vi "NEW数据采集传输系统.vi"() -> ()   [LabVIEW 2016, in "数据传输系统.lvlib"]
uses:
  <vilib>/Averna/Notify Icon/NotifyIcon.llb/BalloonIcon.ctl
  <vilib>/Utility/miscctls.llb/LVPointTypeDef.ctl
  <vilib>/Utility/config.llb/Read Key (String).vi
  <vilib>/Averna/Notify Icon/NotifyIcon.llb/GetSelectedItemEvent.vi
  <vilib>/Averna/Notify Icon/NotifyIcon.llb/SetVisible.vi
  <vilib>/Averna/Notify Icon/NotifyIcon.llb/SetMenuDefaultItem.vi
  <vilib>/Averna/Notify Icon/NotifyIcon.llb/SetTipText.vi
  <vilib>/Utility/config.llb/NI_LVConfig.lvlib
  data/FreeMem.dll
  <vilib>/Averna/Notify Icon/NotifyIcon.llb/NotifyIcon.lvclass
panel:
  out "错误输出":errorcluster
  in  "停止输入":bool caption="停止 2"
  in  "系统编码选择框":string(combo)="地表水质量监测"
  in  "数据发送通道":enum16{"TCP", "VISA"}(ring)
  in  "baud rate":u32=9600 caption="波特率"
  in  "VISA resource name":refnum<visa-resource-name> caption="VISA资源名称"
  in  "实时数据发送时间间隔/min":i32=1
  in  "数据组合发送":bool
  in  "日志、参数发送":bool
  in  "2011发送":bool
  in  "判断数据反馈":bool
  in  "数据发送协议":enum16{"2005-212协议", "2017-212协议"}(ring)=enum."2017-212协议"
  in  "重发时间":T1(ring)
  in  "重发日期":T2(ring)
  in  "开机启动":bool
  in  "确定更改起始时间":bool
  in  "更改起始时间":bool
  in  "数据发送起始时间":timestamp format="%<%.3X\n%Y/%m/%d>T"
  in  "每周自动重发":bool=TRUE
  in  "确定":bool
  in  "返回":bool
  in  "PW":string
  in  "MN":string
  in  "PORT":string
  in  "IP":string
  in  "站点设备":string
  in  "站点名称":string
  out "设置超时时间/min":i32=1
  out "状态信息":T3={"1st Error to Convert "=63, "步骤 "=enum."发送数据", "元素"="实时数据", "TCP服务端掉线计数"=0, "TCP掉线时间节点"="2019/05/08 15:24:17"} {"1st Error to Convert" items=["无错误", "参数错误", "内存已满", "超出区域", "文件结束", "文件已打开", "一般文件IO错误", "未找到文件", "文件权限错误", "磁盘已满", "路径副本", "打开过多文件", "未启用", "未找到资源文件", "无法添加资源", "未找到资源", "未找到图像", "图像内存错误", "画笔不存在", "配置错误类型", "配置未找到解析段", "配置解析错误", "配置内存错误", "错误外部代码格式", "错误外部代码偏移量", "外部代码不存在", "空窗口", "销毁窗口错误", "空菜单", "打印已中止", "错误打印记录", "打印驱动程序错误", "打印时窗口错误", "打印时内存错误", "打印对话框错误", "一般打印错误", "无效设备引用句柄", "设备未找到", "设备参数错误", "设备单位错误", "无法打开设备", "设备调用已中止", "一般错误", "用户已取消", "对象ID过低", "对象ID过高", "对象不在堆中", "未知的堆", "错误DefProc ID", "DefProc不在表格中", "范围外信息", "空方法", "未知信息", "不支持管理器调用", "错误地址", "连接过程中", "连接超时", "连接过程中", "不支持网络属性", "网络错误", "正在使用的地址", "系统缺少内存", "连接已中止", "连接已拒绝", "连接未建立", "连接已建立", "连接已关闭", "初始化错误（交互应用程序管理器）", "错误事件发生", "等待无约束事件发生处理程序", "事件发生队列溢出", "错误路径", "未发出信号量", "未识别类型（交互应用程序管理器）"]}
  out "数据接收超时指示灯":bool
  out "空闲时间/s":string
  out "系统时间":string
  out "实时小时数据上传":bool
  out "系统状态改变":bool
  out "软件版本":string
  out "掉线指示":bool
  out "核查数据上传":bool
  out "配置信息":T4
  in  "参数配置":bool
  out "查询数据发送":bool
  out "读取报文显示":string
  out "发送报文显示":string
  out "心跳包":bool
  out "通信状态":bool
  # "数 据 采 集 传 输 系 统"
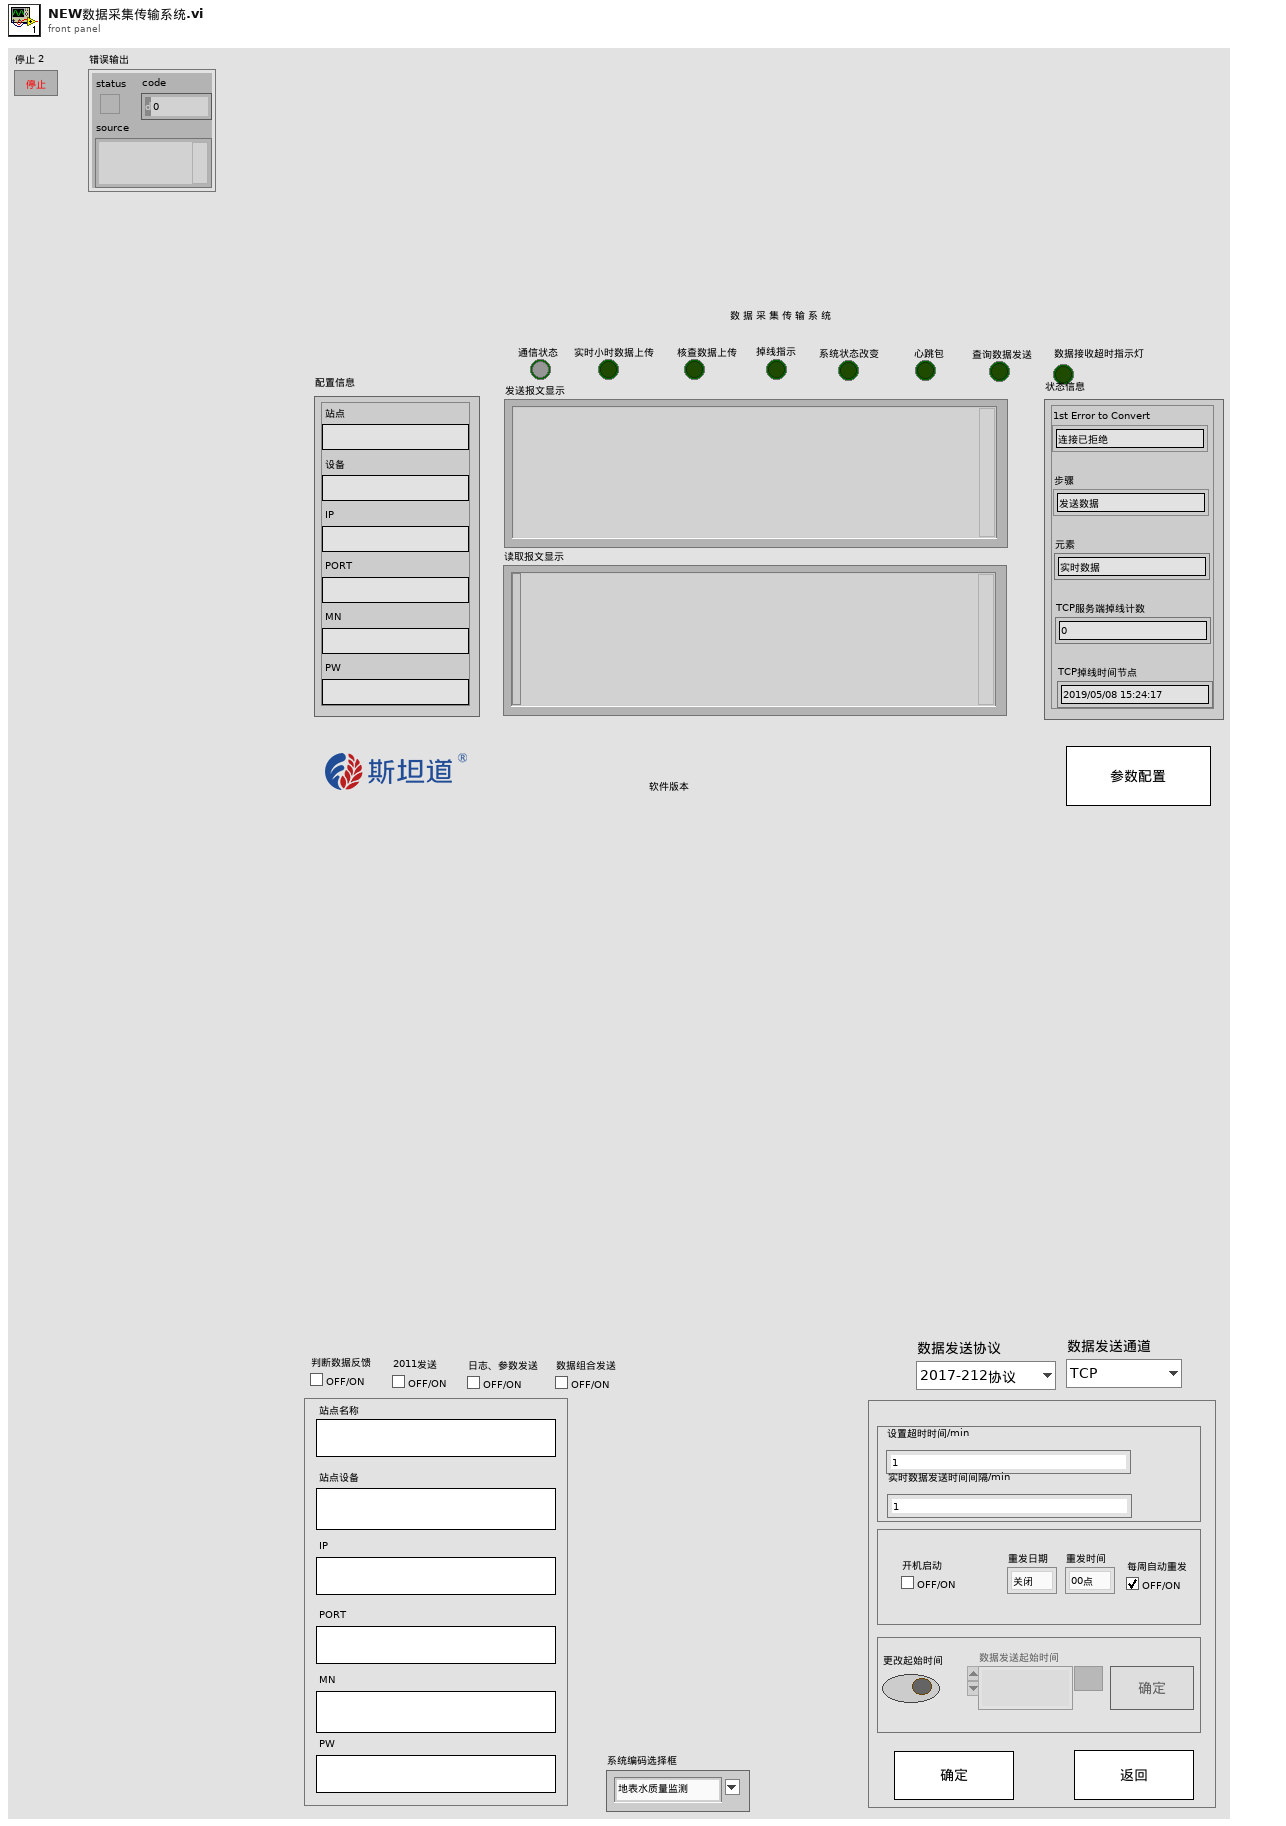
[diagram p1: front panel]
types:
  T1 = enum16{"00点", "01点", "02点", "03点", "04点", "05点", "06点", "07点", "08点", "09点", "10点", "11点", "12点", "13点", "14点", "15点", "16点", "17点", "18点", "19点", "20点", "21点", "22点", "23点"}
  T2 = enum16{"关闭", "星期日", "星期一", "星期二", "星期三", "星期四", "星期五", "星期六"}
  T3 = cluster{"1st Error to Convert ":i32, "步骤 ":enum16{"打开连接", "发送数据", "读取数据", "数据处理", "关闭连接"}, "元素":string, "TCP服务端掉线计数":i32, "TCP掉线时间节点":string}
  T4 = cluster{"站点":string, "设备":string, "IP":string, "PORT":string, "MN":string, "PW":string}
  T5 = enum32{"invalid app kind", "Development System", "Run Time System", "Student Edition", "Embedded LabVIEW", "Evaluation", "Custom"}
  T6 = enum8{"Enabled", "Disabled", "Disabled and Grayed Out"}
  T7 = typedef "LVPointTypeDef.ctl" = cluster{"Horizontal":i16, "Vertical":i16}
  T8 = typedef "imagedata.ctl" = cluster{"image type":i32, "image depth":i32, "image":u8[], "mask":u8[], "colors":u32[], "Rectangle":cluster{"left":i16, "top":i16, "right":i16, "bottom":i16}}
  T9 = typedef "NI_LVConfig.lvlib/Config Data RefNum.ctl" = refnum<k1>
  T10 = cluster{"CODMn":bool, "CODCr":bool, "DO":bool, "铜":bool, "PH":bool, "氨氮":bool, "比电导率":bool, "水温":bool, "盐度(海水)":bool, "浊度":bool, "总氮":bool, "总磷":bool, "叶绿素a":bool, "藻密度":bool, "水位":bool, "流速":bool, "瞬时流量":bool, "累积流量":bool}
  T11 = typedef "LVDateTimeRec.ctl" = cluster{"秒数的小数部分":dbl, "秒":i32, "分":i32, "时":i32, "日":i32, "月":i32, "年":i32, "天数（周）":i32, "天数（年）":i32, "DST":i32}
  T12 = enum32{"Invalid", "Standard", "Closed", "Hidden", "Minimized", "Maximized"}
  T13 = typedef "NotifyIcon.lvlib/NotifyIcon.lvclass/BalloonIcon.ctl" = enum32{"None", "Information", "Warning", "Error"}
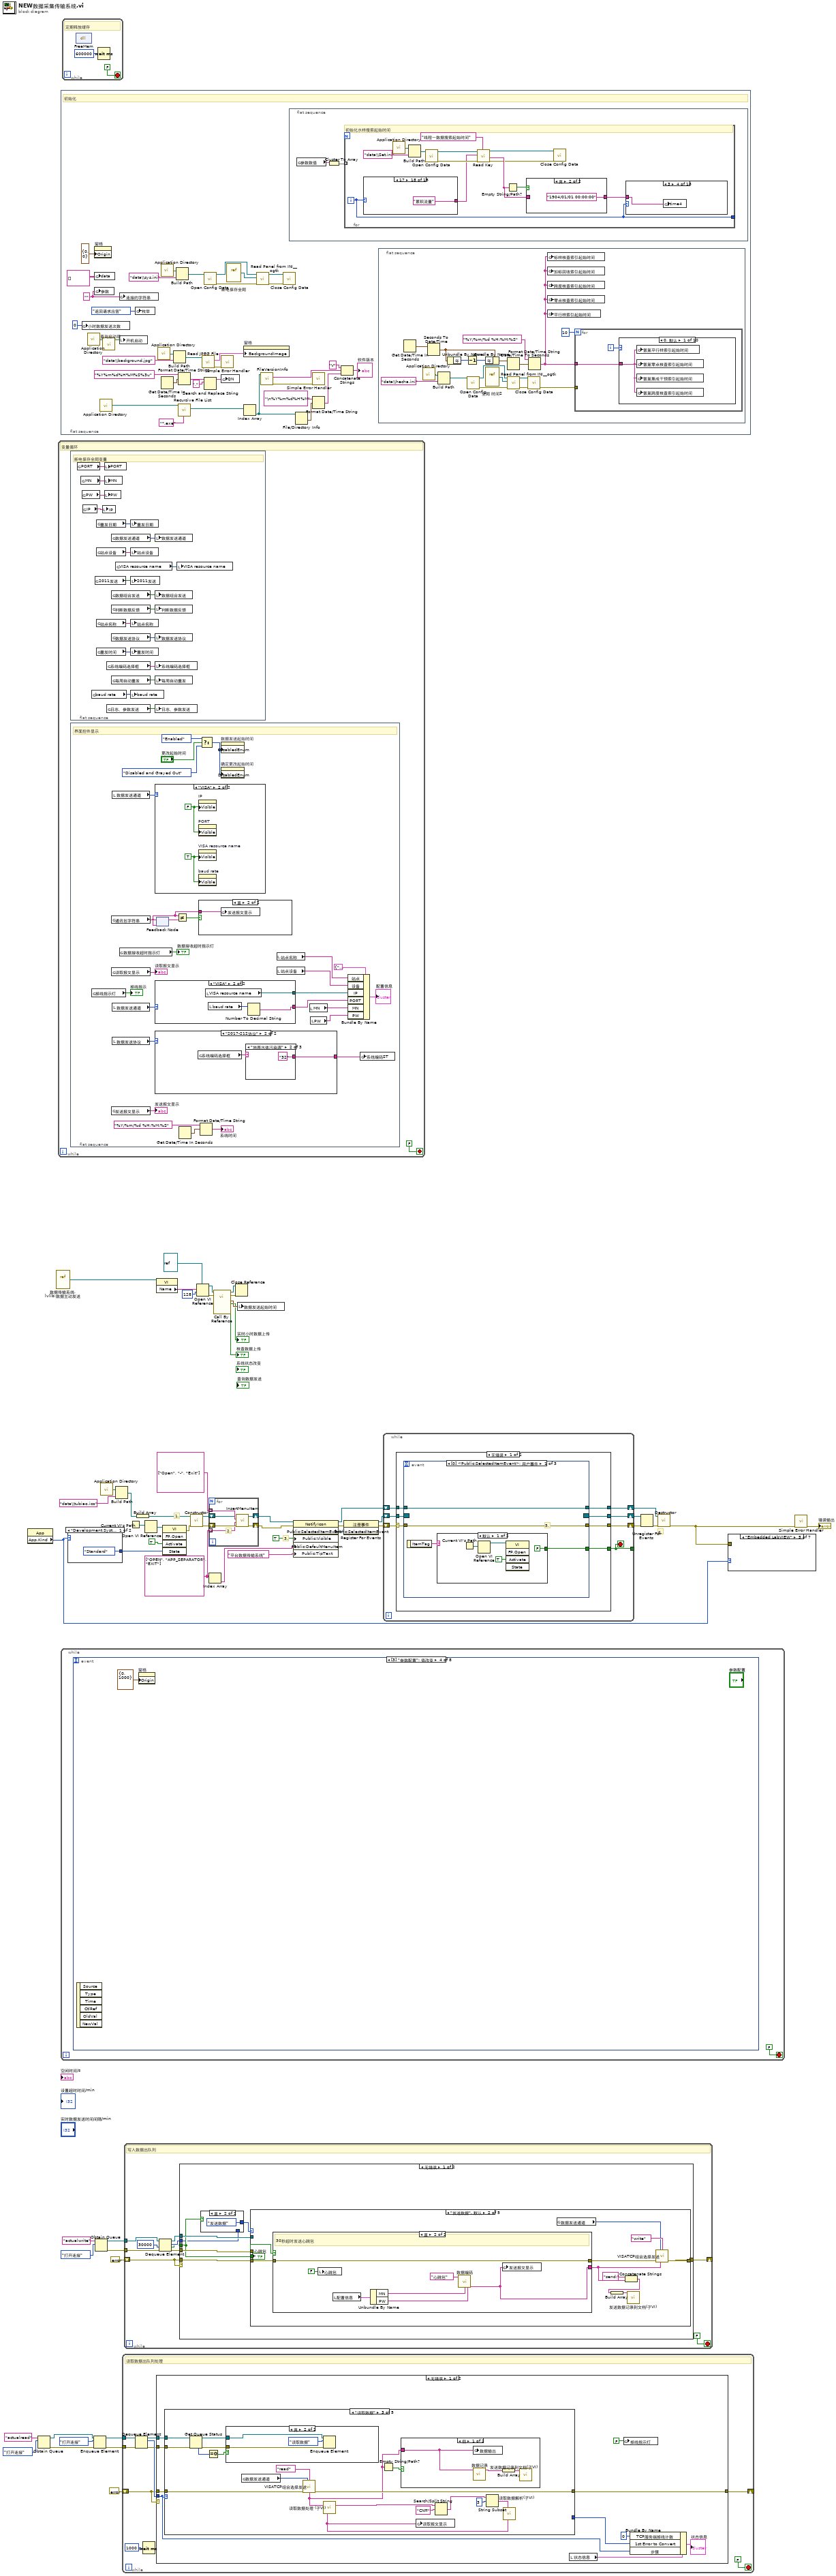
[diagram p0: block diagram]
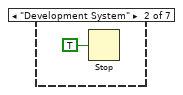
[diagram p3: hidden frame]
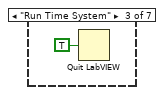
[diagram p4: hidden frame]
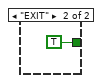
[diagram p8: hidden frame]
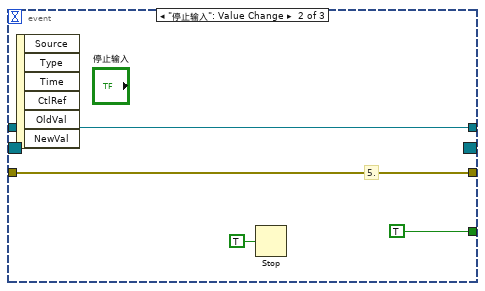
[diagram p9: hidden frame]
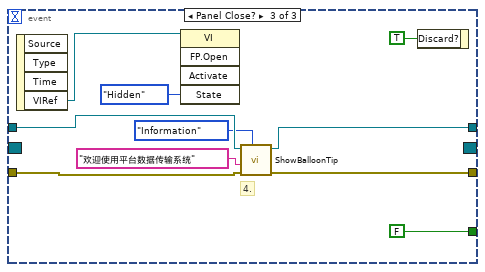
[diagram p10: hidden frame]
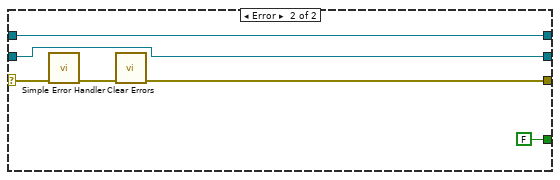
[diagram p11: hidden frame]
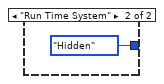
[diagram p12: hidden frame]
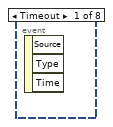
[diagram p13: hidden frame]
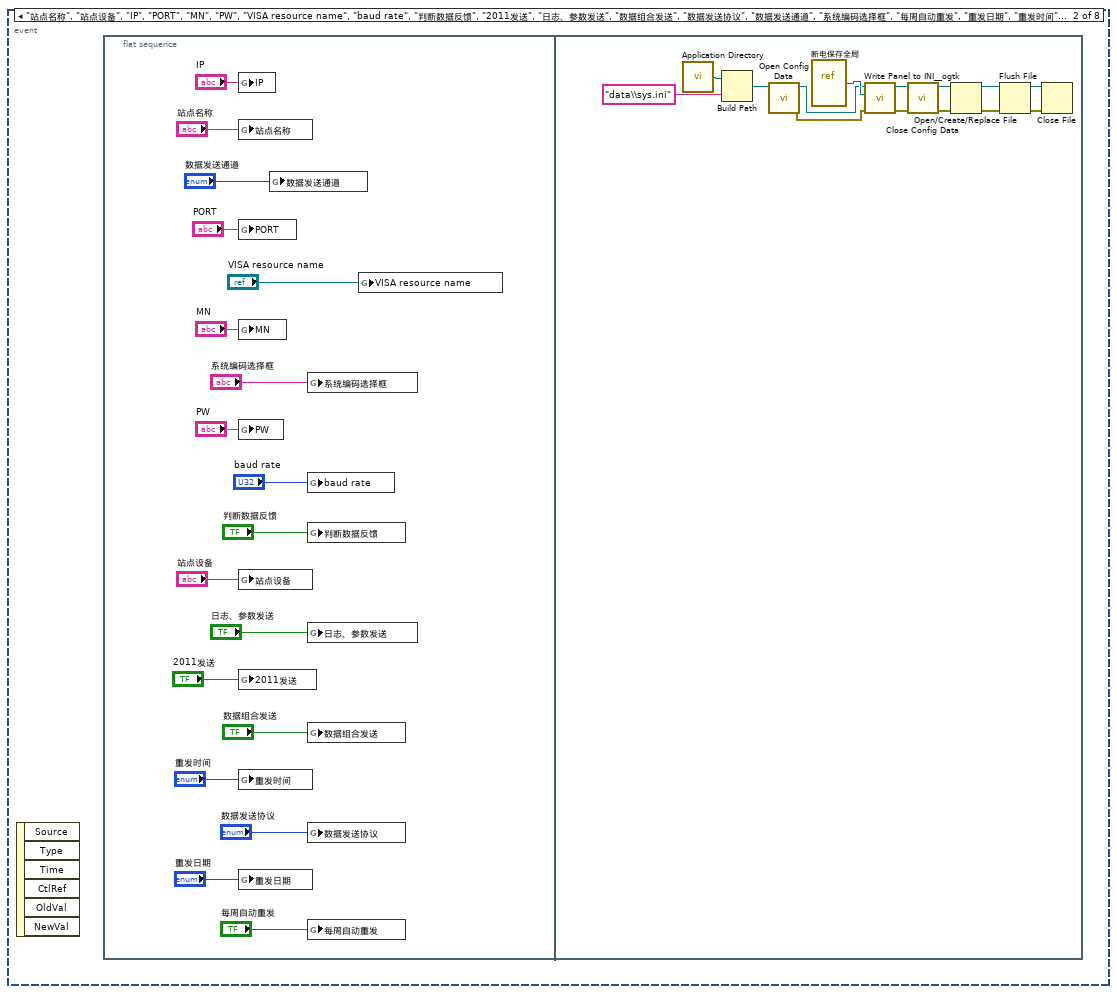
[diagram p14: hidden frame]
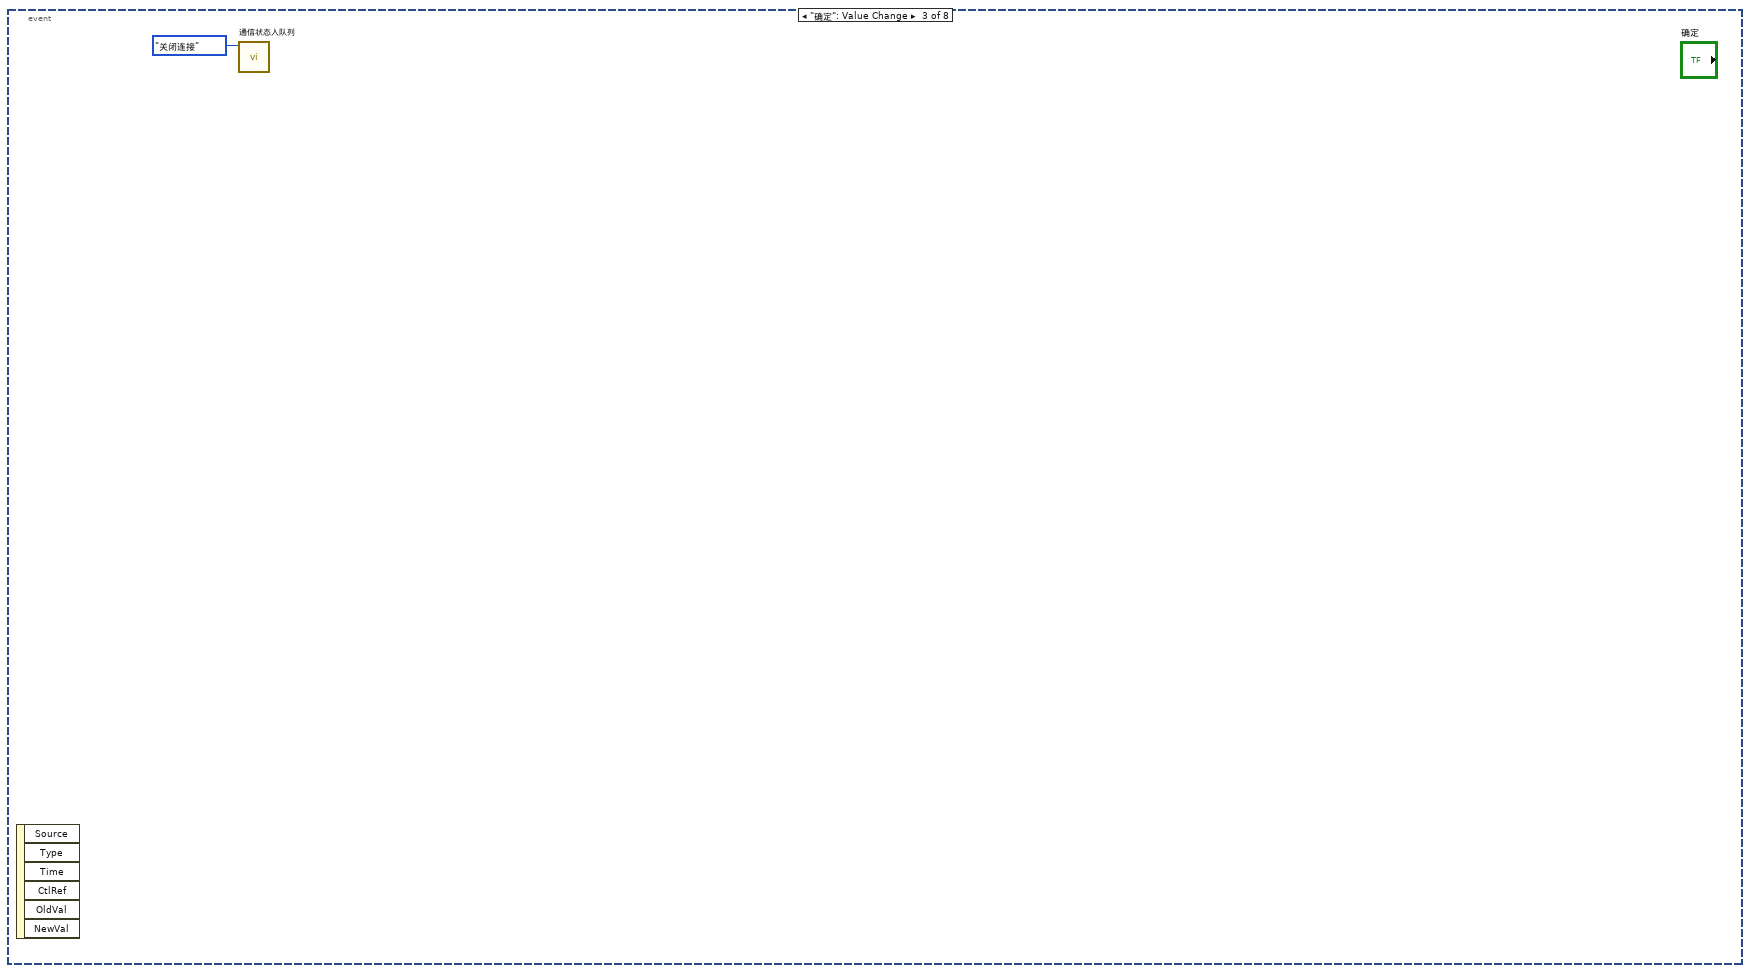
[diagram p15: hidden frame]
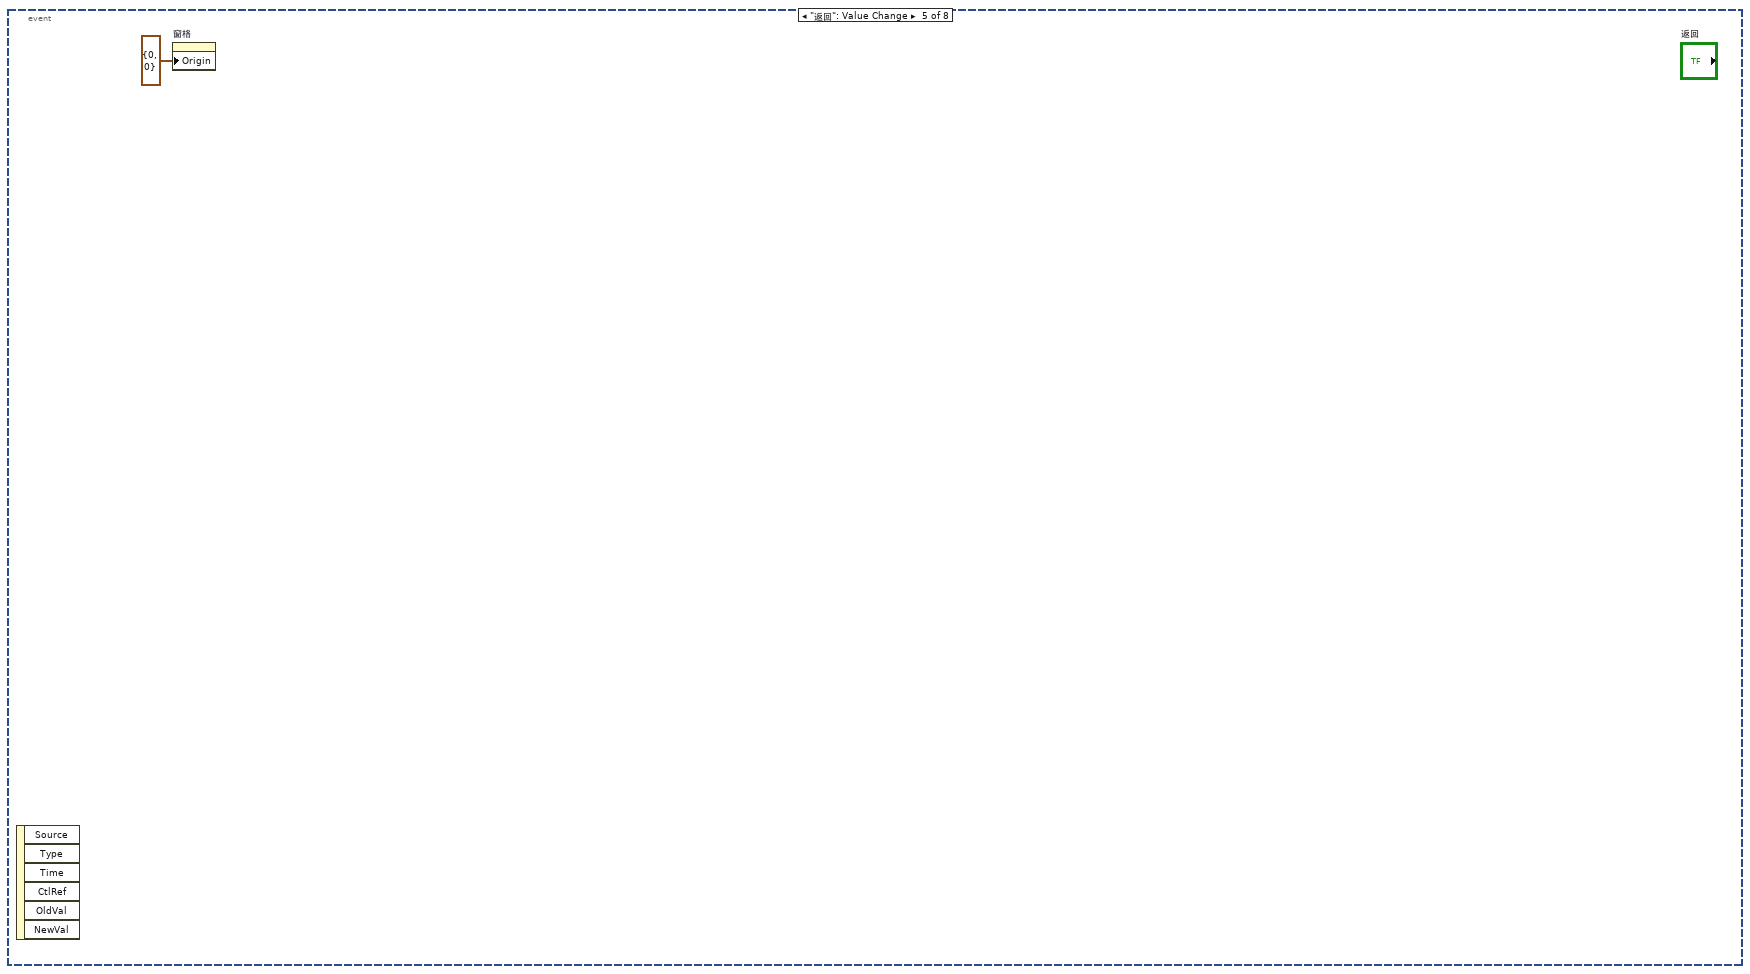
[diagram p16: hidden frame]
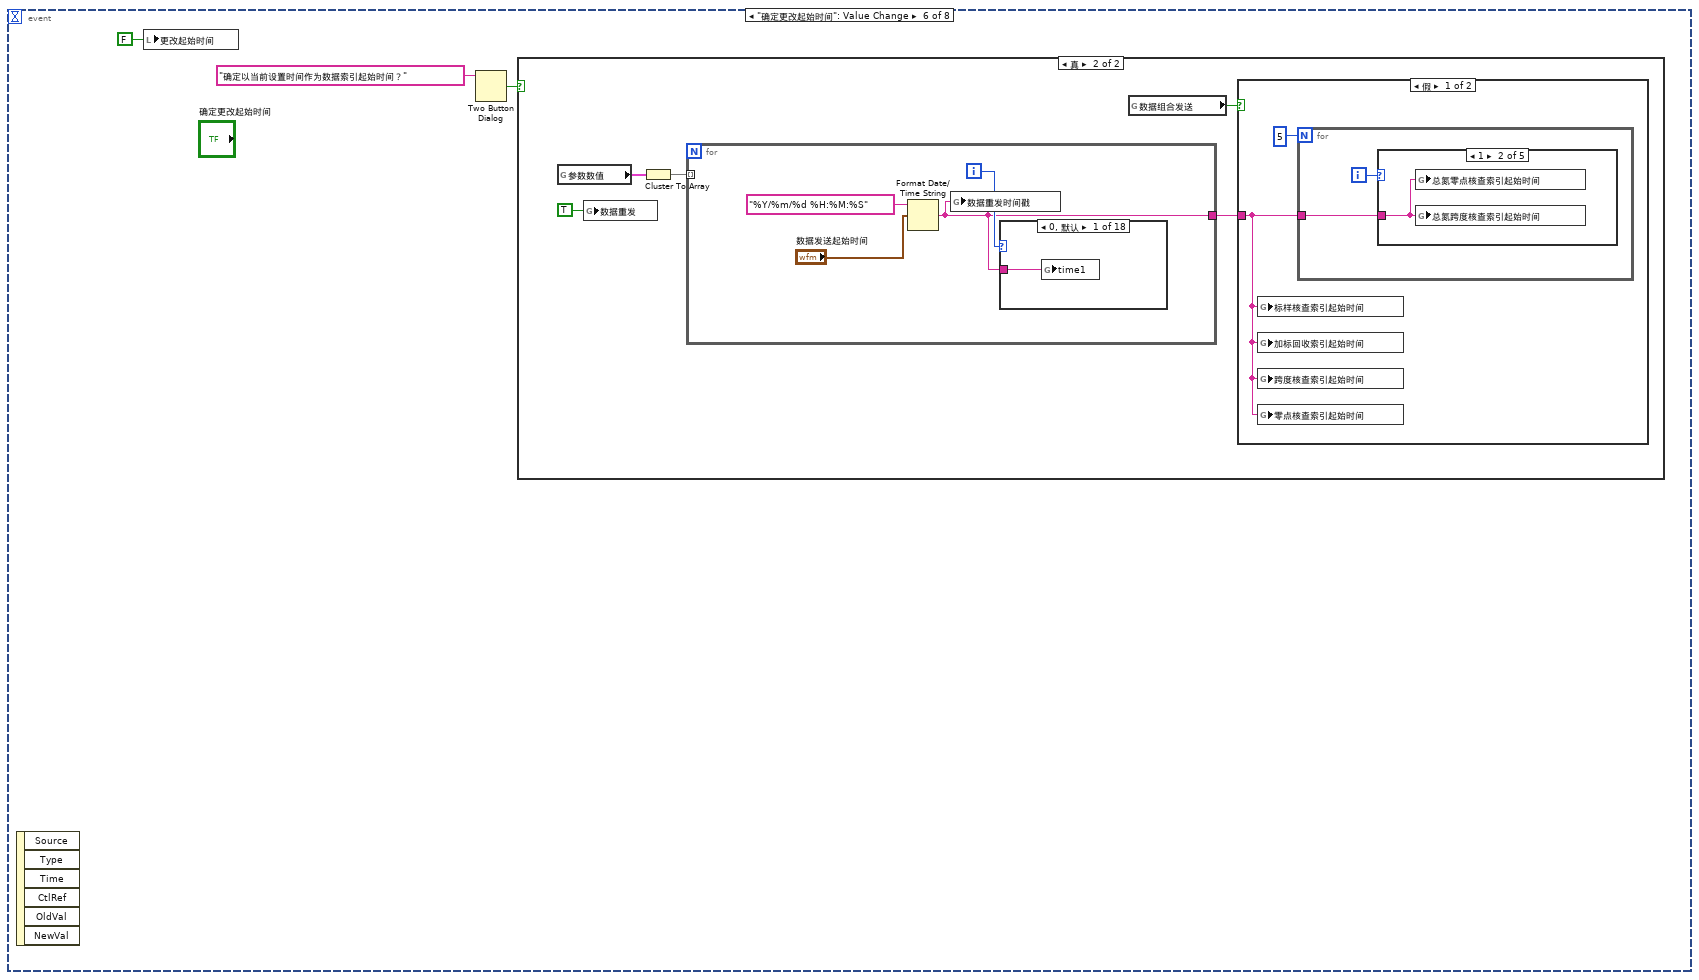
[diagram p17: hidden frame]
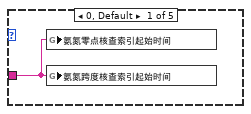
[diagram p19: hidden frame]
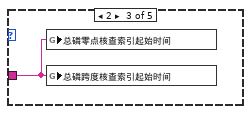
[diagram p20: hidden frame]
diagram:
  w9 = string[] ["OPEN", "APP_SEPARATOR", "EXIT"]
  # "6."
  # "3."
  # "1."
  n1 = property class="App"() -> ("App.Kind"=w1:T5)  [unwired: 2 in, 2 out]
  n2 = Obtain Queue(name (unnamed)="actualread" ("名称（未命名）"), element data type=enum16{"打开连接", "发送数据", "读取数据", "数据处理", "关闭连接"}."打开连接" ("枚举")) -> (queue out=w54:refnum<queue>, error out=w47:errorcluster)  [unwired: 3 in, 1 out]
  n3 = vi-ref "数据传输系统.lvlib:数据主动发送.vi"() -> (w41:refnum<vi>)
  n4 = while {
    stop <- FALSE stop-if-true
    # "变量循环"
    n5 = flat-sequence {
      frame #0 {
        # "断电保存全局变量"
        n6 = global read "断电保存全局.vi" "PORT"() -> (w112:string)
        n7 = global read "断电保存全局.vi" "MN"() -> (w111:string)
        n8 = global read "断电保存全局.vi" "PW"() -> (w110:string)
        n9 = global read "断电保存全局.vi" "IP"() -> (w113:string)
        n10 = global read "断电保存全局.vi" "baud rate"() -> (w108:u32)
        n11 = global read "断电保存全局.vi" "2011发送"() -> (w104:bool)
        n12 = global read "断电保存全局.vi" "重发日期"() -> (w106:T2)
        n13 = global read "断电保存全局.vi" "站点设备"() -> (w114:string)
        n14 = global read "断电保存全局.vi" "站点名称"() -> (w115:string)
        n15 = global read "断电保存全局.vi" "重发时间"() -> (w98:T1)
        n16 = local write "IP"(w113) -> ()
        n17 = local write "PORT"(w112) -> ()
        n18 = local write "MN"(w111) -> ()
        n19 = local write "PW"(w110) -> ()
        n20 = global read "断电保存全局.vi" "系统编码选择框"() -> (w99:string)
        n21 = global read "断电保存全局.vi" "日志、参数发送"() -> (w103:bool)
        n22 = global read "断电保存全局.vi" "数据发送通道"() -> (w100:enum16{"TCP", "VISA"})
        n23 = global read "断电保存全局.vi" "数据组合发送"() -> (w102:bool)
        n24 = global read "断电保存全局.vi" "判断数据反馈"() -> (w105:bool)
        n25 = global read "断电保存全局.vi" "数据发送协议"() -> (w101:enum16{"2005-212协议", "2017-212协议"})
        n26 = global read "断电保存全局.vi" "每周自动重发"() -> (w107:bool)
        n27 = global read "断电保存全局.vi" "VISA resource name"() -> (w109:refnum<visa-resource-name>)
        n28 = local write "重发日期"(w106) -> ()
        n29 = local write "站点设备"(w114) -> ()
        n30 = local write "2011发送"(w104) -> ()
        n31 = local write "站点名称"(w115) -> ()
        n32 = local write "重发时间"(w98) -> ()
        n33 = local write "baud rate"(w108) -> ()
        n34 = local write "数据发送通道"(w100) -> ()
        n35 = local write "数据组合发送"(w102) -> ()
        n36 = local write "判断数据反馈"(w105) -> ()
        n37 = local write "数据发送协议"(w101) -> ()
        n38 = local write "系统编码选择框"(w99) -> ()
        n39 = local write "每周自动重发"(w107) -> ()
        n40 = local write "日志、参数发送"(w103) -> ()
        n41 = local write "VISA resource name"(w109) -> ()
      }
    }
    n42 = flat-sequence {
      frame #0 {
        # "界面控件显示"
        n43 = global read "全局 数据发送重叠.vi" "掉线指示灯"() -> (→"掉线指示":bool)
        n44 = global read "全局1.vi" "通讯包字符串"() -> (w62:string)
        n45 = global read "全局1.vi" "读取报文显示"() -> (→"读取报文显示":string)
        n46 = global read "全局1.vi" "发送报文显示"() -> (→"发送报文显示":string)
        n47 = local read "数据发送通道"() -> (w56:enum16{"TCP", "VISA"})
        n48 = local read "数据发送通道"() -> (w81:enum16{"TCP", "VISA"})
        n49 = local read "数据发送协议"() -> (w70:enum16{"2005-212协议", "2017-212协议"})
        n50 = global read "全局 数据发送重叠.vi" "数据接收超时指示灯"() -> (→"数据接收超时指示灯":bool)
        n51 = case shown="\"VISA\"" w56 {
          frame "TCP", Default {
            w82 = TRUE ("可见")
            w83 = FALSE ("可见")
            n52 = property on="IP" class="Str"("Visible"=w82) -> ()  [unwired: 2 in, 2 out]
            n53 = property on="PORT" class="Str"("Visible"=w82) -> ()  [unwired: 2 in, 2 out]
            n54 = property on="VISA resource name" class="VISAName"("Visible"=w83) -> ()  [unwired: 2 in, 2 out]
            n55 = property on="baud rate" class="DigNum (严格)"("Visible"=w83) -> ()  [unwired: 2 in, 2 out]
          }
          frame "VISA" {
            w84 = FALSE ("可见")
            w85 = TRUE ("可见")
            n56 = property on="IP" class="Str"("Visible"=w84) -> ()  [unwired: 2 in, 2 out]
            n57 = property on="PORT" class="Str"("Visible"=w84) -> ()  [unwired: 2 in, 2 out]
            n58 = property on="VISA resource name" class="VISAName"("Visible"=w85) -> ()  [unwired: 2 in, 2 out]
            n59 = property on="baud rate" class="DigNum (严格)"("Visible"=w85) -> ()  [unwired: 2 in, 2 out]
          }
        }
        n60 = case shown="\"VISA\"" w81 {
          tunnel: [w94 w97] -> w78
          tunnel: [w93 w95] -> w75
          frame "TCP", Default {
            n61 = local read "PORT"() -> (w93:string)
            n62 = local read "IP"() -> (w94:string)
          }
          frame "VISA" {
            n63 = local read "VISA resource name"() -> (w97:refnum<visa-resource-name>)
            n64 = local read "baud rate"() -> (w96:u32)
            n65 = Number To Decimal String(number=w96) -> (decimal integer string=w95:string)  [unwired: 1 in]
          }
        }
        n66 = case shown="\"2017-212协议\"" w70 {
          tunnel: ["32" ("设备编码MN") w88] -> w69
          frame "2005-212协议", Default {
          }
          frame "2017-212协议" {
            n67 = global read "断电保存全局.vi" "系统编码选择框"() -> (w89:string)
            n68 = case shown="\"地表水体污染源\"" w89 {
              tunnel: ["52" ("设备编码MN") "32" ("设备编码MN") "21" ("设备编码MN")] -> w88
              frame "污水排放过程监测" {
              }
              frame "地表水体污染源" {
              }
              frame "地表水质量监测", Default {
              }
            }
          }
        }
        n69 = feedback #1(w62) -> (w63:string)
        n70 = feedback-in #1(w62) -> ()
        n71 = Not Equal?(x=w62, y=w63) -> (x != y?=w61:bool)
        n72 = Get Date/Time In Seconds() -> (seconds since 1Jan1904=w71:timestamp)
        n73 = case shown="真" w61 {
          tunnel: w62 -> [_ w86]
          frame False {
          }
          frame True {
            n74 = global write "全局1.vi" "发送报文显示"(w86) -> ()
          }
        }
        n75 = Format Date/Time String(time format string (%c)="%Y/%m/%d %H:%M:%S" ("时间格式字符串(%c)"), seconds (now)=w71) -> (date/time string=→"系统时间":string)  [unwired: 1 in]
        n76 = Select(t=T6."Enabled" ("禁用"), s="更改起始时间", f=T6."Disabled and Grayed Out" ("禁用")) -> (s? t:f=w57:T6)
        n77 = property on="数据发送起始时间" class="AbsTime (严格)"("DisabledEnum"=w57) -> ()  [unwired: 2 in, 2 out]
        n78 = property on="确定更改起始时间" class="Bool"("DisabledEnum"=w57) -> ()  [unwired: 2 in, 2 out]
        n79 = local read "站点名称"() -> (w77:string)
        n80 = local read "站点设备"() -> (w76:string)
        n81 = local read "MN"() -> (w74:string)
        n82 = local read "PW"() -> (w73:string)
        n83 = Bundle By Name(cluster=T4 {"站点"="", "设备"="", "IP"="", "PORT"="", "MN"="", "PW"=""} ("配置信息"), "站点"=w77, "设备"=w76, "IP"=w78, "PORT"=w75, "MN"=w74, "PW"=w73) -> (→"配置信息":T4)
        n84 = global write "全局1.vi" "系统编码ST"(w69) -> ()
      }
    }
  }
  n85 = flat-sequence {
    frame #0 {
      w149 = "" ("参数")
      # "初始化"
      n86 = global write "全局 小时数据发送次数.vi" "小时数据发送次数"(0 ("数值")) -> ()
      n87 = call <vilib>:"Application Directory.vi"() -> ("Application Directory"=w125:path)
      n88 = property on="窗格" class="Pane"("Origin"=T7 {"Horizontal"=0, "Vertical"=0} ("原点")) -> ()  [unwired: 2 in, 2 out]
      n89 = global write "全局 实时数据参数.vi" "data"(string[][] [] ("data")) -> ()
      n90 = global write "全局 实时数据参数.vi" "参数"(w149) -> ()
      n91 = call <vilib>:"Application Directory.vi"() -> ("Application Directory"=w128:path)
      n92 = call "查询启动项.vi"("启动文件路径"=w125) -> ("包含启动项"=w124:bool)  [unwired: 9 in, 1 out]
      n93 = global write "全局 实时数据参数.vi" "连接的字符串"(w149) -> ()
      n94 = local write "开机启动"(w124) -> ()
      n95 = global write "全局1.vi" "枚举"(enum16{"返回请求应答", "上传数据", "返回执行结果"}."返回请求应答" ("枚举")) -> ()
      n96 = call <vilib>:"Application Directory.vi"() -> ("Application Directory"=w140:path)
      n97 = call <vilib>:"Application Directory.vi"() -> ("Application Directory"=w119:path)
      n98 = Get Date/Time In Seconds() -> (seconds since 1Jan1904=w145:timestamp)
      n99 = Build Path(base path=w140, name or relative path="data\\background.jpg" ("名称或相对路径")) -> (appended path=w139:path)
      n100 = Build Path(base path=w119, name or relative path="data\\sys.ini" ("名称或相对路径")) -> (appended path=w117:path)
      n101 = Format Date/Time String(time format string (%c)="%Y%m%d%H%M%S%3u" ("时间格式字符串(%c)"), seconds (now)=w145) -> (date/time string=w144:string)  [unwired: 1 in]
      n102 = call <vilib>:"Recursive File List.vi"("pattern"="*.exe", "Folder Path"=w128) -> ("All Files in Dir"=w135:path[])  [unwired: 5 in, 4 out]
      n103 = call <vilib>:"Read JPEG File.vi"("path to JPEG file"=w139) -> ("error out"=w137:errorcluster, "image data"=w138:T8)  [unwired: 8 in, 1 out]
      n104 = call <vilib>:"Open Config Data.vi"("configuration file path"=w117) -> ("error out"=w123:errorcluster, "refnum"=w122:T9)  [unwired: 8 in, 1 out]
      n105 = Search and Replace String(input string=w144, search string="." ("搜索字符串")) -> (result string=w142:string)  [unwired: 6 in, 3 out]
      n106 = call <vilib>:"Simple Error Handler.vi"("error in (no error)"=w137) -> ()  [unwired: 4 in, 5 out]
      n107 = global write "全局1.vi" "QN"(w142) -> ()
      n108 = vi-ref "断电保存全局.vi"() -> (w121:refnum<vi>)
      n109 = property on="窗格" class="Pane"("BackgroundImage"=w138) -> ()  [unwired: 2 in, 2 out]
      n110 = Index Array(array=w135) -> (element=w134:path)  [unwired: 1 in]
      n111 = call <userlib>:"Read Panel from INI__ogtk.vi"("error in (no error)"=w123, "VI ref"=w121, "refnum"=w122) -> ("error out"=w116:errorcluster, "refnum out"=w120:T9)  [unwired: 7 in]
      n112 = call <vilib>:"FileVersionInfo.vi"("Application Path in"=w134) -> ("error out"=w127:errorcluster, "File Version Info"=w130:string)  [unwired: 7 in, 2 out]
      n113 = call <vilib>:"Close Config Data.vi"("error in (no error)"=w116, "refnum"=w120) -> ()  [unwired: 8 in, 2 out]
      n114 = flat-sequence {
        frame #0 {
          n115 = global read "全局1.vi" "参数数值"() -> (w152:T10)
          n116 = Cluster To Array(cluster=w152) -> (array=w153:bool[])
          n117 = for {
            tunnel: w153 -> [_] mode=indexing
            tunnel: [w156] -> _
            i -> [w156]
            # "初始化水样搜索起始时间"
            n118 = case shown="17" w156 {
              tunnel: ["CODMn" "CODCr" "DO" "铜" "PH" "氨氮" "比电导率" "水温" "盐度(海水)" "浊度" "总氮" "总磷" "叶绿素a" "藻密度" "水位" "流速" "瞬时流量" "累积流量"] -> w160
              frame 0, Default {
              }
              frame 1 {
              }
              frame 2 {
              }
              frame 3 {
              }
              frame 4 {
              }
              frame 5 {
              }
              frame 6 {
              }
              frame 7 {
              }
              frame 8 {
              }
              frame 9 {
              }
              frame 10 {
              }
              frame 11 {
              }
              frame 12 {
              }
              frame 13 {
              }
              frame 14 {
              }
              frame 15 {
              }
              frame 16 {
              }
              frame 17 {
              }
            }
            n119 = call <vilib>:"Application Directory.vi"() -> ("Application Directory"=w166:path)
            n120 = Build Path(base path=w166, name or relative path="data\\Set.ini" ("名称或相对路径")) -> (appended path=w164:path)
            n121 = call <vilib>:"Open Config Data.vi"("configuration file path"=w164) -> ("error out"=w162:errorcluster, "refnum"=w163:T9)  [unwired: 8 in, 1 out]
            n122 = call-poly <vilib>:"Read Key.vi"("section"="线程一数据搜索起始时间", "error in (no error)"=w162, "key"=w160, "refnum"=w163) -> ("error out"=w154:errorcluster, "value"=w157:string, "refnum out"=w155:T9)  [unwired: 4 in, 1 out]
            n123 = Empty String/Path?(string/path=w157) -> (empty?=w159:bool)
            n124 = case shown="真" w159 {
              tunnel: [w167 "1904/01/01 00:00:00"] -> w158
              tunnel: w157 -> [w167 _]
              frame False {
              }
              frame True {
              }
            }
            n125 = call <vilib>:"Close Config Data.vi"("error in (no error)"=w154, "refnum"=w155) -> ()  [unwired: 8 in, 2 out]
            n126 = case shown="3" w156 {
              tunnel: w158 -> [w169 w170 w171 w172 w173 w174 w175 w176 w177 w178 w179 w180 w181 w182 w183 w184 w185 w186]
              frame 0, Default {
                n127 = global write "全局 水样时间.vi" "time1"(w169) -> ()
              }
              frame 1 {
                n128 = global write "全局 水样时间.vi" "time2"(w170) -> ()
              }
              frame 2 {
                n129 = global write "全局 水样时间.vi" "time3"(w171) -> ()
              }
              frame 3 {
                n130 = global write "全局 水样时间.vi" "time4"(w172) -> ()
              }
              frame 4 {
                n131 = global write "全局 水样时间.vi" "time5"(w173) -> ()
              }
              frame 5 {
                n132 = global write "全局 水样时间.vi" "time6"(w174) -> ()
              }
              frame 6 {
                n133 = global write "全局 水样时间.vi" "time7"(w175) -> ()
              }
              frame 7 {
                n134 = global write "全局 水样时间.vi" "time8"(w176) -> ()
              }
              frame 8 {
                n135 = global write "全局 水样时间.vi" "time9"(w177) -> ()
              }
              frame 9 {
                n136 = global write "全局 水样时间.vi" "time10"(w178) -> ()
              }
              frame 10 {
                n137 = global write "全局 水样时间.vi" "time11"(w179) -> ()
              }
              frame 11 {
                n138 = global write "全局 水样时间.vi" "time12"(w180) -> ()
              }
              frame 12 {
                n139 = global write "全局 水样时间.vi" "time13"(w181) -> ()
              }
              frame 13 {
                n140 = global write "全局 水样时间.vi" "time14"(w182) -> ()
              }
              frame 14 {
                n141 = global write "全局 水样时间.vi" "time15"(w183) -> ()
              }
              frame 15 {
                n142 = global write "全局 水样时间.vi" "time16"(w184) -> ()
              }
              frame 16 {
                n143 = global write "全局 水样时间.vi" "time17"(w185) -> ()
              }
              frame 17 {
                n144 = global write "全局 水样时间.vi" "time18"(w186) -> ()
              }
            }
          }
        }
      }
      n145 = File/Directory Info(path=w134) -> (last mod=w133:timestamp)  [unwired: 1 in, 6 out]
      n146 = call <vilib>:"Simple Error Handler.vi"("error in (no error)"=w127) -> ()  [unwired: 4 in, 5 out]
      n147 = Format Date/Time String(time format string (%c)="\n%Y%m%d%H%M" ("时间格式字符串(%c)"), seconds (now)=w133) -> (date/time string=w129:string)  [unwired: 1 in]
      n148 = Concatenate Strings("V" ("字符串"), w130, w129) -> (→"软件版本":string)
      n149 = flat-sequence {
        frame #0 {
          n150 = Get Date/Time In Seconds() -> (seconds since 1Jan1904=w222:timestamp)
          n151 = call <vilib>:"Application Directory.vi"() -> ("Application Directory"=w212:path)
          n152 = Seconds To Date/Time(time stamp (now)=w222) -> (date time rec=w220:T11)  [unwired: 1 in]
          n153 = Build Path(base path=w212, name or relative path="data\\hecha.ini" ("名称或相对路径")) -> (appended path=w214:path)
          n154 = Unbundle By Name(w220) -> ("年"=w221:i32)
          n155 = Decrement(x=w221) -> (x-1=w219:i32)
          n156 = call <vilib>:"Open Config Data.vi"("configuration file path"=w214) -> ("error out"=w208:errorcluster, "refnum"=w209:T9)  [unwired: 8 in, 1 out]
          n157 = Bundle By Name(cluster=w220, "年"=w219) -> (w217:T11)
          n158 = vi-ref "全局 时间2.vi"() -> (w210:refnum<vi>)
          n159 = Date/Time To Seconds(2:w217) -> (0:w218:timestamp)  [unwired: 1 in]
          n160 = call <userlib>:"Read Panel from INI__ogtk.vi"("error in (no error)"=w208, "VI ref"=w210, "refnum"=w209) -> ("error out"=w207:errorcluster, "refnum out"=w211:T9)  [unwired: 7 in]
          n161 = call <vilib>:"Close Config Data.vi"("error in (no error)"=w207, "refnum"=w211) -> ("error out"=w206:errorcluster)  [unwired: 8 in, 1 out]
          n162 = Format Date/Time String(time format string (%c)="%Y/%m/%d %H:%M:%S" ("时间格式字符串(%c)"), seconds (now)=w218) -> (date/time string=w215:string)  [unwired: 1 in]
          n163 = global write "全局 时间2.vi" "标样核查索引起始时间"(w215) -> ()
          n164 = global write "全局 时间2.vi" "加标回收索引起始时间"(w215) -> ()
          n165 = global write "全局 时间2.vi" "跨度核查索引起始时间"(w215) -> ()
          n166 = global write "全局 时间2.vi" "零点核查索引起始时间"(w215) -> ()
          n167 = global write "全局 时间2.vi" "平行样索引起始时间"(w215) -> ()
          n168 = for {
            N: 10 -> [_]
            tunnel: w215 -> [w223]
            tunnel: w206 -> [_]
            i -> [w224]
            n169 = case shown="0, 默认" w224 {
              tunnel: w223 -> [w225 w226 w227 w228 w229 w230 w231 w232 w233 w234]
              frame 0, Default {
                n170 = global write "全局 时间2.vi" "氨氮平行样索引起始时间"(w225) -> ()
                n171 = global write "全局 时间2.vi" "氨氮零点核查索引起始时间"(w225) -> ()
                n172 = global write "全局 时间2.vi" "氨氮集成干预索引起始时间"(w225) -> ()
                n173 = global write "全局 时间2.vi" "氨氮跨度核查索引起始时间"(w225) -> ()
              }
              frame 1 {
                n174 = global write "全局 时间2.vi" "总氮零点核查索引起始时间"(w226) -> ()
                n175 = global write "全局 时间2.vi" "总氮平行样索引起始时间"(w226) -> ()
                n176 = global write "全局 时间2.vi" "总氮跨度核查索引起始时间"(w226) -> ()
                n177 = global write "全局 时间2.vi" "总氮集成干预索引起始时间"(w226) -> ()
              }
              frame 2 {
                n178 = global write "全局 时间2.vi" "总磷零点核查索引起始时间"(w227) -> ()
                n179 = global write "全局 时间2.vi" "总磷平行样索引起始时间"(w227) -> ()
                n180 = global write "全局 时间2.vi" "总磷跨度核查索引起始时间"(w227) -> ()
                n181 = global write "全局 时间2.vi" "总磷集成干预索引起始时间"(w227) -> ()
              }
              frame 3 {
                n182 = global write "全局 时间2.vi" "CODMn零点核查索引起始时间"(w228) -> ()
                n183 = global write "全局 时间2.vi" "CODMn平行样索引起始时间"(w228) -> ()
                n184 = global write "全局 时间2.vi" "CODMn跨度核查索引起始时间"(w228) -> ()
                n185 = global write "全局 时间2.vi" "CODMn集成干预索引起始时间"(w228) -> ()
              }
              frame 4 {
                n186 = global write "全局 时间2.vi" "CODCr零点核查索引起始时间"(w229) -> ()
                n187 = global write "全局 时间2.vi" "CODCr平行样索引起始时间"(w229) -> ()
                n188 = global write "全局 时间2.vi" "CODCr跨度核查索引起始时间"(w229) -> ()
                n189 = global write "全局 时间2.vi" "CODCr集成干预索引起始时间"(w229) -> ()
              }
              frame 5 {
                n190 = global write "全局 时间2.vi" "DO集成干预索引起始时间"(w230) -> ()
              }
              frame 6 {
                n191 = global write "全局 时间2.vi" "PH集成干预索引起始时间"(w231) -> ()
              }
              frame 7 {
                n192 = global write "全局 时间2.vi" "比电导率集成干预索引起始时间"(w232) -> ()
              }
              frame 8 {
                n193 = global write "全局 时间2.vi" "水温集成干预索引起始时间"(w233) -> ()
              }
              frame 9 {
                n194 = global write "全局 时间2.vi" "浊度集成干预索引起始时间"(w234) -> ()
              }
            }
          }
        }
      }
    }
  }
  n195 = while {
    stop <- FALSE stop-if-true
    n196 = event shown="[3] \"参数配置\": 值改变" {
      selector: _ -> [_ _ _ _ _ _ _ _]
      dyn-events: _ -> [_ _ _ _ _ _ _ _]
      timeout: _ -> [_ _ _ _ _ _ _ _]
      event Timeout {
        n197 = event-data() -> ()  [unwired: 1 in, 3 out]
      }
      event "站点名称", "站点设备", "IP", "PORT", "MN", "PW", "VISA resource name", "baud rate", "判断数据反馈", "2011发送", "日志、参数发送", "数据组合发送", "数据发送协议", "数据发送通道", "系统编码选择框", "每周自动重发", "重发日期", "重发时间": Value Change {
        n198 = event-data() -> ()  [unwired: 1 in, 6 out]
        n199 = flat-sequence {
          frame #0 {
            n200 = global write "断电保存全局.vi" "IP"("IP") -> ()
            n201 = global write "断电保存全局.vi" "站点名称"("站点名称") -> ()
            n202 = global write "断电保存全局.vi" "PORT"("PORT") -> ()
            n203 = global write "断电保存全局.vi" "MN"("MN") -> ()
            n204 = global write "断电保存全局.vi" "PW"("PW") -> ()
            n205 = global write "断电保存全局.vi" "站点设备"("站点设备") -> ()
            n206 = global write "断电保存全局.vi" "2011发送"("2011发送") -> ()
            n207 = global write "断电保存全局.vi" "重发时间"("重发时间") -> ()
            n208 = global write "断电保存全局.vi" "重发日期"("重发日期") -> ()
            n209 = global write "断电保存全局.vi" "数据发送通道"("数据发送通道") -> ()
            n210 = global write "断电保存全局.vi" "系统编码选择框"("系统编码选择框") -> ()
            n211 = global write "断电保存全局.vi" "baud rate"("baud rate") -> ()
            n212 = global write "断电保存全局.vi" "判断数据反馈"("判断数据反馈") -> ()
            n213 = global write "断电保存全局.vi" "日志、参数发送"("日志、参数发送") -> ()
            n214 = global write "断电保存全局.vi" "数据组合发送"("数据组合发送") -> ()
            n215 = global write "断电保存全局.vi" "数据发送协议"("数据发送协议") -> ()
            n216 = global write "断电保存全局.vi" "每周自动重发"("每周自动重发") -> ()
            n217 = global write "断电保存全局.vi" "VISA resource name"("VISA resource name") -> ()
          }
          frame #1 {
            n218 = call <vilib>:"Application Directory.vi"() -> ("Application Directory"=w254:path)
            n219 = Build Path(base path=w254, name or relative path="data\\sys.ini" ("名称或相对路径")) -> (appended path=w256:path)
            n220 = call <vilib>:"Open Config Data.vi"("configuration file path"=w256) -> ("error out"=w260:errorcluster, "refnum"=w257:T9)  [unwired: 8 in, 1 out]
            n221 = vi-ref "断电保存全局.vi"() -> (w258:refnum<vi>)
            n222 = call <userlib>:"Write Panel to INI__ogtk.vi"("error in (no error)"=w260, "VI ref"=w258, "refnum"=w257) -> ("error out"=w261:errorcluster, "refnum out"=w259:T9)  [unwired: 7 in]
            n223 = call <vilib>:"Close Config Data.vi"("error in (no error)"=w261, "refnum"=w259) -> ("error out"=w266:errorcluster, "file path"=w267:path)  [unwired: 8 in]
            n224 = Open/Create/Replace File(file path (use dialog)=w267, error in=w266) -> (refnum out=w263:refnum<file>, error out=w262:errorcluster)  [unwired: 4 in, 1 out]
            n225 = Flush File(refnum=w263, error in=w262) -> (refnum out=w264:refnum<file>, error out=w265:errorcluster)
            n226 = Close File(refnum=w264, error in=w265) -> ()  [unwired: 2 out]
          }
        }
      }
      event "确定": Value Change {
        n227 = event-data() -> ()  [unwired: 1 in, 6 out]
        n228 = call "通信状态入队列.vi"("枚举"=enum16{"打开连接", "发送数据", "读取数据", "数据处理", "关闭连接"}."关闭连接") -> ()  [unwired: 10 in, 1 out]
      }
      event "参数配置": Value Change {
        n229 = event-data() -> ()  [unwired: 1 in, 6 out]
        n230 = property on="窗格" class="Pane"("Origin"=T7 {"Horizontal"=0, "Vertical"=1000} ("原点")) -> ()  [unwired: 2 in, 2 out]
      }
      event "返回": Value Change {
        n231 = event-data() -> ()  [unwired: 1 in, 6 out]
        n232 = property on="窗格" class="Pane"("Origin"=T7 {"Horizontal"=0, "Vertical"=0} ("原点")) -> ()  [unwired: 2 in, 2 out]
      }
      event "确定更改起始时间": Value Change {
        n233 = event-data() -> ()  [unwired: 1 in, 6 out]
        n234 = local write "更改起始时间"(FALSE ("更改起始时间")) -> ()
        n235 = Two Button Dialog(message="确定以当前设置时间作为数据索引起始时间？" ("消息")) -> (T button?=w271:bool)  [unwired: 2 in]
        n236 = case shown="真" w271 {
          frame False {
          }
          frame True {
            n237 = global read "全局1.vi" "参数数值"() -> (w274:T10)
            n238 = global write "断电保存全局.vi" "数据重发"(TRUE ("数据重发")) -> ()
            n239 = Cluster To Array(cluster=w274) -> (array=w278:bool[])
            n240 = for {
              tunnel: w278 -> [_] mode=indexing
              tunnel: [w289] -> w277
              i -> [w290]
              n241 = Format Date/Time String(time format string (%c)="%Y/%m/%d %H:%M:%S" ("时间格式字符串(%c)"), seconds (now)="数据发送起始时间") -> (date/time string=w289:string)  [unwired: 1 in]
              n242 = global write "断电保存全局.vi" "数据重发时间戳"(w289) -> ()
              n243 = case shown="0, 默认" w290 {
                tunnel: w289 -> [w292 w293 w294 w295 w296 w297 w298 w299 w300 w301 w302 w303 w304 w305 w306 w307 w308 w309]
                frame 0, Default {
                  n244 = global write "全局 水样时间.vi" "time1"(w292) -> ()
                }
                frame 1 {
                  n245 = global write "全局 水样时间.vi" "time2"(w293) -> ()
                }
                frame 2 {
                  n246 = global write "全局 水样时间.vi" "time3"(w294) -> ()
                }
                frame 3 {
                  n247 = global write "全局 水样时间.vi" "time4"(w295) -> ()
                }
                frame 4 {
                  n248 = global write "全局 水样时间.vi" "time5"(w296) -> ()
                }
                frame 5 {
                  n249 = global write "全局 水样时间.vi" "time6"(w297) -> ()
                }
                frame 6 {
                  n250 = global write "全局 水样时间.vi" "time7"(w298) -> ()
                }
                frame 7 {
                  n251 = global write "全局 水样时间.vi" "time8"(w299) -> ()
                }
                frame 8 {
                  n252 = global write "全局 水样时间.vi" "time9"(w300) -> ()
                }
                frame 9 {
                  n253 = global write "全局 水样时间.vi" "time10"(w301) -> ()
                }
                frame 10 {
                  n254 = global write "全局 水样时间.vi" "time11"(w302) -> ()
                }
                frame 11 {
                  n255 = global write "全局 水样时间.vi" "time12"(w303) -> ()
                }
                frame 12 {
                  n256 = global write "全局 水样时间.vi" "time13"(w304) -> ()
                }
                frame 13 {
                  n257 = global write "全局 水样时间.vi" "time14"(w305) -> ()
                }
                frame 14 {
                  n258 = global write "全局 水样时间.vi" "time15"(w306) -> ()
                }
                frame 15 {
                  n259 = global write "全局 水样时间.vi" "time16"(w307) -> ()
                }
                frame 16 {
                  n260 = global write "全局 水样时间.vi" "time17"(w308) -> ()
                }
                frame 17 {
                  n261 = global write "全局 水样时间.vi" "time18"(w309) -> ()
                }
              }
            }
            n262 = global read "断电保存全局.vi" "数据组合发送"() -> (w275:bool)
            n263 = case shown="假" w275 {
              tunnel: w277 -> [w279 _]
              frame False {
                n264 = global write "全局 时间2.vi" "标样核查索引起始时间"(w279) -> ()
                n265 = global write "全局 时间2.vi" "加标回收索引起始时间"(w279) -> ()
                n266 = global write "全局 时间2.vi" "跨度核查索引起始时间"(w279) -> ()
                n267 = global write "全局 时间2.vi" "零点核查索引起始时间"(w279) -> ()
                n268 = for {
                  N: 5 -> [_]
                  tunnel: w279 -> [w281]
                  i -> [w282]
                  n269 = case shown="1" w282 {
                    tunnel: w281 -> [w283 w284 w285 w286 w287]
                    frame 0, Default {
                      n270 = global write "全局 时间2.vi" "氨氮零点核查索引起始时间"(w283) -> ()
                      n271 = global write "全局 时间2.vi" "氨氮跨度核查索引起始时间"(w283) -> ()
                    }
                    frame 1 {
                      n272 = global write "全局 时间2.vi" "总氮零点核查索引起始时间"(w284) -> ()
                      n273 = global write "全局 时间2.vi" "总氮跨度核查索引起始时间"(w284) -> ()
                    }
                    frame 2 {
                      n274 = global write "全局 时间2.vi" "总磷零点核查索引起始时间"(w285) -> ()
                      n275 = global write "全局 时间2.vi" "总磷跨度核查索引起始时间"(w285) -> ()
                    }
                    frame 3 {
                      n276 = global write "全局 时间2.vi" "CODMn零点核查索引起始时间"(w286) -> ()
                      n277 = global write "全局 时间2.vi" "CODMn跨度核查索引起始时间"(w286) -> ()
                    }
                    frame 4 {
                      n278 = global write "全局 时间2.vi" "CODCr零点核查索引起始时间"(w287) -> ()
                      n279 = global write "全局 时间2.vi" "CODCr跨度核查索引起始时间"(w287) -> ()
                    }
                  }
                }
              }
              frame True {
              }
            }
          }
        }
      }
      event "开机启动": Value Change {
        n280 = event-data() -> ("NewVal"=w310:bool)  [unwired: 1 in, 5 out]
        n281 = case shown="假" w310 {
          frame False {
            n282 = Two Button Dialog(message="是否删除开机启动" ("消息"), 1:"否" ("F按钮名称（“取消”）"), 2:"是" ("T按钮名称（“确定”）")) -> (T button?=w311:bool)
            n283 = case shown="真" w311 {
              frame False {
              }
              frame True {
                n284 = call <vilib>:"Application Directory.vi"() -> ("Application Directory"=w316:path)
                n285 = call "删除启动项.vi"("启动文件路径"=w316) -> ("删除标记"=w315:bool)  [unwired: 9 in, 1 out]
                n286 = case shown="假" w315 {
                  tunnel: ["删除开机启动失败" ("T按钮名称（“确定”）") "删除开机启动成功" ("T按钮名称（“确定”）")] -> w317
                  frame False {
                  }
                  frame True {
                  }
                }
                n287 = One Button Dialog(message=w317) -> ()  [unwired: 1 in, 1 out]
              }
            }
          }
          frame True {
            n288 = Two Button Dialog(message="是否添加开机启动" ("消息"), 1:"否" ("F按钮名称（“取消”）"), 2:"是" ("T按钮名称（“确定”）")) -> (T button?=w320:bool)
            n289 = case shown="真" w320 {
              frame False {
              }
              frame True {
                n290 = call <vilib>:"Application Directory.vi"() -> ("Application Directory"=w326:path)
                n291 = call "添加启动项.vi"("启动文件路径"=w326) -> ("添加成功标记"=w325:bool)  [unwired: 9 in, 1 out]
                n292 = case shown="真" w325 {
                  tunnel: ["添加开机启动失败" ("T按钮名称（“确定”）") "添加开机启动成功" ("T按钮名称（“确定”）")] -> w324
                  frame False {
                  }
                  frame True {
                  }
                }
                n293 = One Button Dialog(message=w324) -> ()  [unwired: 1 in, 1 out]
              }
            }
          }
        }
      }
      event "IP", "PORT": Mouse Down {
        n294 = event-data() -> ("CtlRef"=w332:refnum<vi>)  [unwired: 1 in, 7 out]
        n295 = property class="Str"(reference=w332) -> (reference out=w330:refnum<vi>, "Value"=w331:string)  [unwired: 1 in, 1 out]
        n296 = call "IP键盘.vi"("OldNumber"=w331) -> ("NewNumber"=w329:string)
        n297 = property class="Str"(reference=w330, "Val(Sgnl)"=w329) -> ()  [unwired: 1 in, 2 out]
      }
    }
  }
  n298 = while {
    stop <- FALSE stop-if-true
    # "定期释放缓存"
    n299 = dll-call lib="PTH2habs D\tgitkrakenMy softwarecc0平台数采程序 - V1.0.1（修改迭代版）dataFreeMem.dll" fn="FreeMem"() -> ()  [unwired: 4 in, 2 out]
    n300 = Wait (ms)(milliseconds to wait=u32 600000 ("等待时间（毫秒）")) -> ()  [unwired: 1 out]
  }
  n301 = case shown="\"Development System\", 默认" w1 {
    tunnel: [T12."Standard" ("状态") T12."Hidden" ("状态")] -> w28
    frame "Development System", Default {
    }
    frame "Run Time System" {
    }
  }
  n302 = Enqueue Element(queue=w54, element=enum16{"打开连接", "发送数据", "读取数据", "数据处理", "关闭连接"}."打开连接" ("枚举"), error in (no error)=w47) -> (queue out=w50:refnum<queue>, error out=w49:errorcluster)  [unwired: 1 in, 1 out]
  n303 = Obtain Queue(name (unnamed)="actualwrite" ("名称（未命名）"), element data type=enum16{"打开连接", "发送数据", "读取数据", "数据处理", "关闭连接"}."打开连接" ("枚举")) -> (queue out=w44:refnum<queue>, error out=w43:errorcluster)  [unwired: 3 in, 1 out]
  n304 = call <vilib>:"Application Directory.vi"() -> ("Application Directory"=w7:path)
  n305 = Build Path(base path=w7, name or relative path="data\\tubiao.ico" ("名称或相对路径")) -> (appended path=w17:path)
  n306 = while {
    tunnel: w50 -> [w345]
    tunnel: w49 -> [w344]
    shift-right: [w341] -> _
    shift-left: errorcluster {"status"=FALSE, "code"=0, "source"=""} ("error out") -> [w340]
    stop <- FALSE stop-if-true
    # "读取数据出队列处理"
    n307 = Dequeue Element(queue=w345, error in (no error)=w344) -> (queue out=w339:refnum<queue>, element=w342:enum16{"打开连接", "发送数据", "读取数据", "数据处理", "关闭连接"}, error out=w338:errorcluster)  [unwired: 1 in, 1 out]
    n308 = Wait (ms)(milliseconds to wait=u32 1000 ("等待时间（毫秒）")) -> ()  [unwired: 1 out]
    n309 = case shown="无错误" w340 {
      tunnel: w342 -> [w348 _]
      tunnel: [w355 w402] -> w341
      tunnel: w340 -> [w354 w406]
      tunnel: w339 -> [w353 w404]
      tunnel: w338 -> [w352 w403]
      frame No Error {
        n310 = case shown="\"读取数据\"" w348 {
          tunnel: [w361 _ w384 _ w397] -> w355
          tunnel: w354 -> [w360 _ w387 _ w398]
          tunnel: w353 -> [w358 _ w377 _ w395]
          tunnel: w352 -> [w357 _ w376 _ w394]
          tunnel: [w356 _ _ _ _] -> w349
          frame "打开连接", Default {
            n311 = Enqueue Element(queue=w358, element=enum16{"打开连接", "发送数据", "读取数据", "数据处理", "关闭连接"}."读取数据" ("枚举"), error in (no error)=w357) -> ()  [unwired: 1 in, 3 out]
            n312 = global read "断电保存全局.vi" "VISA resource name"() -> (w369:refnum<visa-resource-name>)
            n313 = global read "断电保存全局.vi" "数据发送通道"() -> (w366:enum16{"TCP", "VISA"})
            n314 = global read "断电保存全局.vi" "baud rate"() -> (w368:u32)
            n315 = global read "断电保存全局.vi" "PORT"() -> (w367:string)
            n316 = global read "断电保存全局.vi" "IP"() -> (w365:string)
            n317 = call "VISATCP组合选择发送.vi"("IP"=w365, "数据发送通道"=w366, "命令"="open", "PORT"=w367, "VISA resource name"=w369, "baud rate"=w368, "error in (no error)"=w360) -> ("错误输出"=w361:errorcluster)  [unwired: 5 in, 3 out]
            n318 = Unbundle By Name(w361) -> ("status"=w362:bool, "code"=w356:i32)
            n319 = Not(x=w362) -> (.not. x?=→"通信状态":bool)
          }
          frame "发送数据" {
          }
          frame "读取数据" {
            n320 = Get Queue Status(queue=w377, error in (no error)=w376) -> (queue out=w373:refnum<queue>, error out=w372:errorcluster, # elements in queue=w375:i32)  [unwired: 1 in, 5 out]
            n321 = Equal To 0?(x=w375) -> (x = 0?=w374:bool)
            n322 = case shown="真" w374 {
              tunnel: w373 -> [_ w392]
              tunnel: w372 -> [_ w391]
              frame False {
              }
              frame True {
                n323 = Enqueue Element(queue=w392, element=enum16{"打开连接", "发送数据", "读取数据", "数据处理", "关闭连接"}."读取数据" ("枚举"), error in (no error)=w391) -> ()  [unwired: 1 in, 3 out]
              }
            }
            n324 = global read "断电保存全局.vi" "数据发送通道"() -> (w386:enum16{"TCP", "VISA"})
            n325 = call "VISATCP组合选择发送.vi"("数据发送通道"=w386, "命令"="read", "error in (no error)"=w387) -> ("读取缓冲区"=w370:string, "错误输出"=w384:errorcluster)  [unwired: 9 in, 2 out]
            n326 = call "读取数据处理 (子VI).vi"("data out"=w370) -> ("命令编码CN"=w380:string, "数据"=w378:string)  [unwired: 8 in, 5 out]
            n327 = Empty String/Path?(string/path=w370) -> (empty?=w371:bool)
            n328 = case shown="假" w371 {
              tunnel: w370 -> [w390 _]
              frame False {
                n329 = global write "全局1.vi" "数据输出"(w390) -> ()
                n330 = call "数据记录.vi"("写入字段"=w390) -> ("连接的字符串"=w388:string)  [unwired: 10 in]
                n331 = Build Array(w388) -> (w389:string[])
                n332 = call "发送数据记录到文档(子VI).vi"("数组"=w389) -> ()  [unwired: 9 in, 1 out]
              }
              frame True {
              }
            }
            n333 = global write "全局1.vi" "读取报文显示"(w378) -> ()
            n334 = Search/Split String(string=w380, search string/char (-)="CN=" ("搜索字符串/字符(-)")) -> (match + rest of string=w381:string)  [unwired: 1 in, 2 out]
            n335 = String Subset(string=w381, offset (0)=3 ("偏移量(0)")) -> (substring=w379:string)  [unwired: 1 in]
            n336 = call "读取数据解析(子VI).vi"("数据"=w378, "命令编码CN"=w379) -> ()  [unwired: 5 in, 5 out]
          }
          frame "数据处理" {
          }
          frame "关闭连接" {
            n337 = global read "断电保存全局.vi" "数据发送通道"() -> (w400:enum16{"TCP", "VISA"})
            n338 = Enqueue Element(queue=w395, element=enum16{"打开连接", "发送数据", "读取数据", "数据处理", "关闭连接"}."打开连接" ("枚举"), error in (no error)=w394) -> ()  [unwired: 1 in, 3 out]
            n339 = call "VISATCP组合选择发送.vi"("数据发送通道"=w400, "命令"="close", "error in (no error)"=w398) -> ("错误输出"=w399:errorcluster)  [unwired: 9 in, 3 out]
            n340 = call <vilib>:"Clear Errors.vi"("error in (no error)"=w399) -> ("error out"=w397:errorcluster)  [unwired: 5 in, 1 out]
          }
        }
        n341 = local read "状态信息"() -> (w351:T3)
        n342 = global write "全局 数据发送重叠.vi" "掉线指示灯"(FALSE ("掉线指示灯")) -> ()
        n343 = Bundle By Name(cluster=w351, "TCP服务端掉线计数"=0, "1st Error to Convert"=w349, "步骤"=w348) -> (→"状态信息":T3)
      }
      frame Error {
        n344 = Unbundle By Name(w406) -> ("code"=w405:i32)
        n345 = case shown="56" w405 {
          tunnel: w404 -> [w414 w431 w442]
          tunnel: w403 -> [w413 w430 w441]
          tunnel: [w411 w427 w440] -> w402
          frame 0, Default {
            n346 = Flush Queue(queue=w414, error in (no error)=w413) -> (queue out=w416:refnum<queue>, error out=w417:errorcluster)  [unwired: 1 out]
            n347 = local read "状态信息"() -> (w410:T3)
            n348 = global write "全局 数据发送重叠.vi" "掉线指示灯"(TRUE ("掉线指示灯")) -> ()
            n349 = Unbundle By Name(w410) -> ("TCP服务端掉线计数"=w408:i32)
            n350 = Enqueue Element(queue=w416, element=enum16{"打开连接", "发送数据", "读取数据", "数据处理", "关闭连接"}."关闭连接" ("枚举"), error in (no error)=w417) -> (error out=w418:errorcluster)  [unwired: 1 in, 2 out]
            n351 = Increment(x=w408) -> (x+1=w409:i32)
            n352 = Bundle By Name(cluster=w410, "TCP服务端掉线计数"=w409) -> (w407:T3)
            n353 = local write "状态信息"(w407) -> ()
            n354 = call <vilib>:"Clear Errors.vi"("error in (no error)"=w418) -> ("error out"=w411:errorcluster)  [unwired: 5 in, 1 out]
          }
          frame 54, 63 {
            n355 = Flush Queue(queue=w431, error in (no error)=w430) -> (queue out=w433:refnum<queue>, error out=w434:errorcluster)  [unwired: 1 out]
            n356 = local read "状态信息"() -> (w422:T3)
            n357 = global write "全局 数据发送重叠.vi" "掉线指示灯"(TRUE ("掉线指示灯")) -> ()
            n358 = Unbundle By Name(w422) -> ("TCP服务端掉线计数"=w426:i32, "TCP掉线时间节点"=w419:string)
            n359 = Enqueue Element(queue=w433, element=enum16{"打开连接", "发送数据", "读取数据", "数据处理", "关闭连接"}."关闭连接" ("枚举"), error in (no error)=w434) -> (error out=w428:errorcluster)  [unwired: 1 in, 2 out]
            n360 = Less Or Equal?(x=w426, y=1) -> (x <= y?=w424:bool)
            n361 = case shown="真" w424 {
              tunnel: [w435 w436] -> w423
              tunnel: w419 -> [w435 _]
              frame False {
              }
              frame True {
                n362 = Get Date/Time In Seconds() -> (seconds since 1Jan1904=w437:timestamp)
                n363 = Format Date/Time String(time format string (%c)="%Y%m%d%H%M%S%3u" ("时间格式字符串(%c)"), seconds (now)=w437) -> (date/time string=w439:string)  [unwired: 1 in]
                n364 = call "格式时间字符串.vi"("字符串"=w439) -> ("连接的字符串"=w436:string)  [unwired: 10 in]
              }
            }
            n365 = Increment(x=w426) -> (x+1=w421:i32)
            n366 = call <vilib>:"Clear Errors.vi"("error in (no error)"=w428) -> ("error out"=w427:errorcluster)  [unwired: 5 in, 1 out]
            n367 = Bundle By Name(cluster=w422, "TCP服务端掉线计数"=w421, "TCP掉线时间节点"=w423) -> (w420:T3)
            n368 = local write "状态信息"(w420) -> ()
          }
          frame 56 {
            n369 = Flush Queue(queue=w442, error in (no error)=w441) -> (queue out=w444:refnum<queue>, error out=w445:errorcluster)  [unwired: 1 out]
            n370 = Enqueue Element(queue=w444, element=enum16{"打开连接", "发送数据", "读取数据", "数据处理", "关闭连接"}."读取数据" ("枚举"), error in (no error)=w445) -> (error out=w446:errorcluster)  [unwired: 1 in, 2 out]
            n371 = call <vilib>:"Clear Errors.vi"("error in (no error)"=w446) -> ("error out"=w440:errorcluster)  [unwired: 5 in, 1 out]
          }
        }
      }
    }
  }
  n372 = while {
    tunnel: w44 -> [w455]
    tunnel: w43 -> [w454]
    shift-right: [w450] -> _
    shift-left: errorcluster {"status"=FALSE, "code"=0, "source"=""} ("error out") -> [w449]
    stop <- FALSE stop-if-true
    # "写入数据出队列"
    n373 = Dequeue Element(queue=w455, timeout in ms (-1)=30000 ("超时毫秒(-1)"), error in (no error)=w454) -> (queue out=w448:refnum<queue>, element=w452:enum16{"打开连接", "发送数据", "读取数据", "数据处理", "关闭连接"}, timed out?=w451:bool, error out=w447:errorcluster)
    n374 = case shown="无错误" w449 {
      tunnel: w452 -> [w457 _]
      tunnel: w451 -> [w459 _]
      tunnel: [w463 w503] -> w450
      tunnel: w449 -> [w462 w507]
      tunnel: w448 -> [w461 w505]
      tunnel: w447 -> [w460 w504]
      frame No Error {
        n375 = case shown="真" w459 {
          tunnel: [w464 enum16{"打开连接", "发送数据", "读取数据", "数据处理", "关闭连接"}."发送数据" ("枚举")] -> w458
          tunnel: w457 -> [w464 _]
          frame False {
          }
          frame True {
          }
        }
        n376 = case shown="\"发送数据\", 默认" w458 {
          tunnel: w459 -> [_ w480 _ _ _]
          tunnel: [w466 w483 _ _ w496] -> w463
          tunnel: w462 -> [w468 w482 _ _ w497]
          tunnel: w461 -> [_ _ _ _ w498]
          tunnel: w460 -> [_ _ _ _ w495]
          frame "打开连接" {
            n377 = global read "断电保存全局.vi" "VISA resource name"() -> (w475:refnum<visa-resource-name>)
            n378 = global read "断电保存全局.vi" "数据发送通道"() -> (w472:enum16{"TCP", "VISA"})
            n379 = global read "断电保存全局.vi" "baud rate"() -> (w474:u32)
            n380 = global read "断电保存全局.vi" "PORT"() -> (w473:string)
            n381 = global read "断电保存全局.vi" "IP"() -> (w471:string)
            n382 = call "VISATCP组合选择发送.vi"("IP"=w471, "数据发送通道"=w472, "命令"="open", "PORT"=w473, "VISA resource name"=w475, "baud rate"=w474, "error in (no error)"=w468) -> ("错误输出"=w466:errorcluster)  [unwired: 5 in, 3 out]
            n383 = Unbundle By Name(w466) -> ("status"=w469:bool)  [unwired: 1 out]
            n384 = Not(x=w469) -> (.not. x?=w467:bool)
            n385 = local write "通信状态"(w467) -> ()
          }
          frame "发送数据", Default {
            n386 = case shown="真" w480 {
              tunnel: [w487 w489] -> w477
              tunnel: w482 -> [w486 w490]
              tunnel: [w486 w490] -> w481
              frame False {
                # "事件触发发送数据"
                n387 = global read "全局1.vi" "发送报文显示"() -> (w487:string)
              }
              frame True {
                # "30秒超时发送心跳包"
                n388 = local write "心跳包"(FALSE ("心跳包")) -> ()
                n389 = local read "配置信息"() -> (w493:T4)
                n390 = Unbundle By Name(w493) -> ("MN"=w492:string, "PW"=w491:string)
                n391 = call "数据编码.vi"("table输入"="心跳包", "MN"=w492, "PW"=w491) -> ("通讯包字符串"=w489:string)  [unwired: 11 in, 1 out]
                n392 = global write "全局1.vi" "发送报文显示"(w489) -> ()
              }
            }
            n393 = global read "断电保存全局.vi" "数据发送通道"() -> (w484:enum16{"TCP", "VISA"})
            n394 = Concatenate Strings("send:" ("字符串"), w477) -> (w476:string)
            n395 = Build Array(w476) -> (w479:string[])
            n396 = call "发送数据记录到文档(子VI).vi"("数组"=w479) -> ()  [unwired: 9 in, 1 out]
            n397 = call "VISATCP组合选择发送.vi"("数据发送通道"=w484, "命令"="write", "error in (no error)"=w481, "写入缓冲区"=w477) -> ("错误输出"=w483:errorcluster)  [unwired: 8 in, 3 out]
            "心跳包" <- w480
          }
          frame "读取数据" {
          }
          frame "数据处理" {
          }
          frame "关闭连接" {
            n398 = global read "断电保存全局.vi" "数据发送通道"() -> (w500:enum16{"TCP", "VISA"})
            n399 = Enqueue Element(queue=w498, element=enum16{"打开连接", "发送数据", "读取数据", "数据处理", "关闭连接"}."打开连接" ("枚举"), error in (no error)=w495) -> ()  [unwired: 1 in, 3 out]
            n400 = call "VISATCP组合选择发送.vi"("数据发送通道"=w500, "命令"="close", "error in (no error)"=w497) -> ("错误输出"=w501:errorcluster)  [unwired: 9 in, 3 out]
            n401 = call <vilib>:"Clear Errors.vi"("error in (no error)"=w501) -> ("error out"=w496:errorcluster)  [unwired: 5 in, 1 out]
          }
        }
      }
      frame Error {
        n402 = Unbundle By Name(w507) -> ("code"=w506:i32)
        n403 = case shown="56" w506 {
          tunnel: w505 -> [w515 w532 w544]
          tunnel: w504 -> [w514 w531 w543]
          tunnel: [w512 w528 w542] -> w503
          frame 0, Default {
            n404 = Flush Queue(queue=w515, error in (no error)=w514) -> (queue out=w517:refnum<queue>, error out=w518:errorcluster)  [unwired: 1 out]
            n405 = local read "状态信息"() -> (w511:T3)
            n406 = global write "全局 数据发送重叠.vi" "掉线指示灯"(TRUE ("掉线指示灯")) -> ()
            n407 = Unbundle By Name(w511) -> ("TCP服务端掉线计数"=w509:i32)
            n408 = Enqueue Element(queue=w517, element=enum16{"打开连接", "发送数据", "读取数据", "数据处理", "关闭连接"}."关闭连接" ("枚举"), error in (no error)=w518) -> (error out=w519:errorcluster)  [unwired: 1 in, 2 out]
            n409 = Increment(x=w509) -> (x+1=w510:i32)
            n410 = Bundle By Name(cluster=w511, "TCP服务端掉线计数"=w510) -> (w508:T3)
            n411 = local write "状态信息"(w508) -> ()
            n412 = call <vilib>:"Clear Errors.vi"("error in (no error)"=w519) -> ("error out"=w512:errorcluster)  [unwired: 5 in, 1 out]
          }
          frame 54, 63 {
            n413 = Flush Queue(queue=w532, error in (no error)=w531) -> (queue out=w534:refnum<queue>, error out=w535:errorcluster)  [unwired: 1 out]
            n414 = local read "状态信息"() -> (w523:T3)
            n415 = global write "全局 数据发送重叠.vi" "掉线指示灯"(TRUE ("掉线指示灯")) -> ()
            n416 = Unbundle By Name(w523) -> ("TCP服务端掉线计数"=w527:i32, "TCP掉线时间节点"=w520:string)
            n417 = Enqueue Element(queue=w534, element=enum16{"打开连接", "发送数据", "读取数据", "数据处理", "关闭连接"}."关闭连接" ("枚举"), error in (no error)=w535) -> (error out=w529:errorcluster)  [unwired: 1 in, 2 out]
            n418 = Less Or Equal?(x=w527, y=1) -> (x <= y?=w525:bool)
            n419 = case shown="真" w525 {
              tunnel: [w536 w537] -> w524
              tunnel: w520 -> [w536 _]
              frame False {
              }
              frame True {
                n420 = Get Date/Time In Seconds() -> (seconds since 1Jan1904=w538:timestamp)
                n421 = Format Date/Time String(time format string (%c)="%Y%m%d%H%M%S%3u" ("时间格式字符串(%c)"), seconds (now)=w538) -> (date/time string=w540:string)  [unwired: 1 in]
                n422 = call "格式时间字符串.vi"("字符串"=w540) -> ("连接的字符串"=w537:string)  [unwired: 10 in]
              }
            }
            n423 = Increment(x=w527) -> (x+1=w522:i32)
            n424 = call <vilib>:"Clear Errors.vi"("error in (no error)"=w529) -> ("error out"=w528:errorcluster)  [unwired: 5 in, 1 out]
            n425 = Bundle By Name(cluster=w523, "TCP服务端掉线计数"=w522, "TCP掉线时间节点"=w524) -> (w521:T3)
            n426 = local write "状态信息"(w521) -> ()
          }
          frame 56 {
            n427 = Flush Queue(queue=w544, error in (no error)=w543) -> (error out=w541:errorcluster)  [unwired: 2 out]
            n428 = call <vilib>:"Clear Errors.vi"("error in (no error)"=w541) -> ("error out"=w542:errorcluster)  [unwired: 5 in, 1 out]
          }
        }
      }
    }
  }
  n429 = Current VI's Path() -> (path=w4:path)
  n430 = Build Array(w17) -> (w12:path[])
  n431 = Open VI Reference(vi path=w4) -> (vi reference=w3:refnum<vi>)  [unwired: 5 in, 1 out]
  n432 = property class="VI"(reference=w41) -> ("Name"=w40:string)  [unwired: 1 in, 2 out]
  n433 = invoke class="VI" method="FP.Open"(reference=w3, "Activate"=TRUE ("激活？"), "State"=w28) -> (error out=w2:errorcluster)  [unwired: 2 in, 4 out]
  n434 = call <vilib>:"Constructor.vi"("error in"=w2, "IconFilePathList"=w12) -> ("error out"=w16:errorcluster, "NotifyIcon"=w8:refnum<class "NotifyIcon.lvclass">)  [unwired: 8 in]
  n435 = Open VI Reference(type specifier VI Refnum (for type only)=refnum<vi> refnum, vi path=w40, options=128 ("选项")) -> (vi reference=w38:refnum<vi>, error out=w36:errorcluster)  [unwired: 3 in]
  n436 = for {
    shift-right: [w549] -> w30
    shift-left: w16 -> [w550]
    tunnel: string[] ["Open", "-", "Exit"] -> [w548] mode=indexing
    tunnel: w9 -> [w547] mode=indexing
    shift-right: [w545] -> w29
    shift-left: w8 -> [w546]
    # "2."
    n437 = call <vilib>:"InsertMenuItem.vi"("error in"=w550, "ItemTag"=w547, "ItemName"=w548, "NotifyIcon in"=w546) -> ("error out"=w549:errorcluster, "NotifyIcon out"=w545:refnum<class "NotifyIcon.lvclass">)  [unwired: 6 in]
  }
  n438 = Index Array(array=w9) -> (element=w10:string)  [unwired: 1 in]
  n439 = call-by-ref "?"(reference=w38, error in=w36) -> (reference out=w34:refnum<vi>, error out=w35:errorcluster, "核查数据上传"=→"核查数据上传":bool, "实时小时数据上传"=→"实时小时数据上传":bool, "数据发送起始时间"=w33:timestamp)  [unwired: 9 in]
  n440 = Close Reference(reference=w34, error in (no error)=w35) -> ()  [unwired: 1 out]
  n441 = local write "数据发送起始时间"(w33) -> ()
  n442 = property class="NotifyIcon"(reference=w29, error in=w30, "Public:Visible"=TRUE ("Visible"), "Public:DefaultMenuItem"=w10, "Public:TipText"="平台数据传输系统" ("TipText")) -> (reference out=w24:refnum<class "NotifyIcon.lvclass">, error out=w15:errorcluster, "Public:SelectedItemEvent"=w14:refnum<user-event>)
  n443 = register-events(error in=w15, w14) -> (reference out=w25:refnum<event-registration>, error out=w26:errorcluster)  [unwired: 1 in]
  n444 = while {
    shift-right: [w554] -> w22
    shift-left: w26 -> [w553]
    shift-right: [w555] -> w19
    shift-left: w24 -> [w556]
    shift-right: [w552] -> w20
    shift-left: w25 -> [w557]
    tunnel: [w551] -> _
    stop <- w551 stop-if-true
    n445 = case shown="无错误" w553 {
      selector: w553 -> [w559 w593]
      tunnel: w557 -> [w564 w588]
      tunnel: w556 -> [w563 w589]
      tunnel: [w562 w589] -> w555
      tunnel: [w561 w591] -> w554
      tunnel: [w560 FALSE ("Discard?")] -> w551
      tunnel: [w558 w588] -> w552
      frame No Error {
        n446 = event shown="[0] <Public:SelectedItemEvent>: 用户事件" {
          selector: w564 -> [_ _ _]
          dyn-events: [_ _ _] -> w558
          timeout: _ -> [_ _ _]
          tunnel: w559 -> [w567 w577 w586]
          tunnel: [w567 w577 w585] -> w561
          tunnel: [w566 TRUE FALSE ("Discard?")] -> w560
          tunnel: w563 -> [w565 w575 w587]
          tunnel: [w565 w575 w584] -> w562
          event User Event {
            # "5."
            n447 = event-data() -> ("ItemTag"=w568:string)  [unwired: 1 in]
            n448 = case shown="默认" w568 {
              tunnel: [FALSE TRUE] -> w566
              frame Default {
                n449 = Current VI's Path() -> (path=w569:path)
                n450 = Open VI Reference(vi path=w569) -> (vi reference=w570:refnum<vi>)  [unwired: 5 in, 1 out]
                n451 = invoke class="VI" method="FP.Open"(reference=w570, "Activate"=TRUE ("激活？")) -> ()  [unwired: 3 in, 5 out]
              }
              frame "EXIT" {
              }
            }
          }
          event "停止输入": Value Change {
            # "5."
            n452 = event-data() -> ()  [unwired: 1 in, 6 out]
            n453 = Stop(stop? (T)=TRUE ("可见")) -> ()
          }
          event Panel Close? {
            # "4."
            n454 = event-data() -> ("VIRef"=w580:refnum<vi>)  [unwired: 1 in, 3 out]
            n455 = invoke class="VI" method="FP.Open"(reference=w580, "State"=T12."Hidden" ("状态")) -> ()  [unwired: 3 in, 5 out]
            n456 = call <vilib>:"ShowBalloonTip.vi"("Balloon Icon"=BalloonIcon."Information", "error in"=w586, "Text"="欢迎使用平台数据传输系统", "NotifyIcon in"=w587) -> ("error out"=w585:errorcluster, "NotifyIcon out"=w584:refnum<class "NotifyIcon.lvclass">)  [unwired: 6 in]
            n457 = event-data("Discard?"=TRUE ("放弃？")) -> ()  [unwired: 1 in, 1 out]
          }
        }
      }
      frame Error {
        n458 = call <vilib>:"Simple Error Handler.vi"("error in (no error)"=w593) -> ("error out"=w592:errorcluster)  [unwired: 4 in, 4 out]
        n459 = call <vilib>:"Clear Errors.vi"("error in (no error)"=w592) -> ("error out"=w591:errorcluster)  [unwired: 5 in, 1 out]
      }
    }
  }
  n460 = Unregister For Events(event registration refnum=w20, error in=w22) -> (error out=w23:errorcluster)
  n461 = call <vilib>:"Destructor.vi"("error in"=w23, "NotifyIcon"=w19) -> ("error out"=w18:errorcluster)  [unwired: 9 in]
  n462 = case shown="\"Embedded LabVIEW\"" w1 {
    tunnel: w18 -> [_ _ _ _ _ _ _]
    frame "invalid app kind", Default {
    }
    frame "Development System" {
      n463 = Stop(stop? (T)=TRUE ("可见")) -> ()
    }
    frame "Run Time System" {
      n464 = Quit LabVIEW(quit? (T)=TRUE ("退出？(T)")) -> ()
    }
    frame "Student Edition" {
    }
    frame "Embedded LabVIEW" {
    }
    frame "Evaluation" {
    }
    frame "Custom" {
    }
  }
  n465 = call <vilib>:"Simple Error Handler.vi"("error in (no error)"=w18) -> ("error out"=→"错误输出":errorcluster)  [unwired: 4 in, 4 out]
